vi "real time object finder single cam 4 way v2.0 EJA 09 16 2016.vi"() -> ()   [LabVIEW 2011]
doc: "The Low-Level Grab VI acquires images continuously and displays the images in an image control using low-level acquisition VIs. A grab is appropriate for high-speed applications in which you need to process only one image at a time."
uses:
  <vilib>/userdefined/High Color/IMAQdx.ctl
  <vilib>/vision/driver/IMAQdx.llb/IMAQdx Buffer Number Mode.ctl
  <vilib>/Utility/file.llb/Write To Spreadsheet File (DBL).vi
  <vilib>/vision/driver/NI_Vision_Acquisition_Software.lvlib
  resource/objmgr/imaqdx.rc
  <vilib>/Analysis/NI_AALBase.lvlib
panel:
  in  "Rectangle":T1
  in  "fish size":i32=200
  out "y position histogram":T2(graph)={"X Values"=[105.75, 139.25, 172.75, 206.25, 239.75, 273.25, 306.75, 340.25, 373.75, 407.25], "Histogram: h(x)"=[42, 48, 50, 100, 118, 231, 514, 357, 278, 63]}
  out "x position histogram":T2(graph)={"X Values"=[76.55, 127.65, 178.75, 229.85, 280.95, 332.05, 383.15, 434.25, 485.35, 536.45], "Histogram: h(x)"=[290, 347, 167, 210, 194, 230, 130, 100, 97, 36]}
  in  "histogram \nbins":i32=10
  in  "always save\non stop\nimaging":bool=TRUE
  in  "acquisition \ntime (s)":i32=60
  in  "save for a \ndesignated \nperiod":bool=TRUE
  out "trajectory":cluster{i32[], i32[]}(graph)
  in  "save\nlast\nimage":bool=TRUE
  in  "stop no save":bool
  out "date stub assigned":string="_2016Y_09M_16D_16h_23m_14s"
  in  "Acquire\ndata":bool
  in  "Experimental stub":string="danio01_test"
  out "Saving":bool
  in  "save data":bool
  in  "save path":path=path "E:/danio_tracking_2016/danio01_09_14_2016"
  in  "number\nformat (%.6f)":string="%.6f"
  in  "Marker\nText color":u32(colorbox)=16711680
  out "Multiplot":cluster{cluster{dbl, i32}[]}[](graph)=[{[{0.0, 251}, {0.034, 257}, {0.067, 266}, {0.1, 275}, {0.133, 283}, {0.167, 294}, {0.201, 308}, {0.234, 321}, {0.267, 332}, {0.3, 340}, {0.333, 346}, {0.367, 349}, {0.401, 351}, {0.434, 351}, {0.467, 350}, {0.5, 349}, {0.534, 350}, {0.567, 351}, {0.601, 352}, {0.634, 351}, {0.667, 351}, {0.701, 351}, {0.734, 350}, {0.767, 346}, {0.8, 343}, {0.833, 337}, {0.867, 331}, {0.901, 326}, {0.934, 322}, {0.967, 317}, {1.0, 314}, {1.034, 309}, {1.067, 304}, {1.1, 301}, {1.134, 298}, {1.167, 295}, {1.201, 291}, {1.234, 287}, {1.267, 282}, {1.3, 276}, {1.333, 269}, {1.367, 262}, {1.401, 258}, {1.434, 255}, {1.467, 252}, {1.5, 247}, {1.534, 244}, {1.567, 241}, {1.6, 238}, {1.633, 235}, {1.666, 232}, {1.701, 229}, {1.734, 227}, {1.767, 225}, {1.8, 222}, {1.833, 221}, {1.867, 220}, {1.9, 220}, {1.933, 220}, {1.967, 218}, {2.0, 219}, {2.034, 219}, {2.067, 217}, {2.1, 215}, {2.133, 216}, {2.166, 217}, {2.201, 220}, {2.234, 227}, {2.267, 238}, {2.3, 250}, {2.333, 261}, {2.367, 274}, {2.4, 283}, {2.434, 288}, {2.467, 294}, {2.5, 297}, {2.534, 297}, {2.567, 299}, {2.6, 302}, {2.633, 306}, {2.666, 313}, {2.701, 321}, {2.734, 330}, {2.767, 339}, {2.8, 348}, {2.833, 355}, {2.867, 364}, {2.901, 372}, {2.934, 380}, {2.967, 388}, {3.0, 395}, {3.034, 404}, {3.067, 412}, {3.101, 419}, {3.134, 427}, {3.167, 433}, {3.201, 441}, {3.234, 447}, {3.267, 453}, {3.3, 459}, {3.333, 463}, {3.368, 468}, {3.401, 472}, {3.434, 477}, {3.467, 483}, {3.5, 490}, {3.534, 496}, {3.567, 505}, {3.6, 512}, {3.634, 516}, {3.667, 521}, {3.701, 524}, {3.734, 524}, {3.767, 522}, {3.8, 521}, {3.833, 518}, {3.868, 513}, {3.901, 509}, {3.934, 504}, {3.967, 499}, {4.0, 495}, {4.034, 489}, {4.068, 482}, {4.101, 478}, {4.134, 476}, {4.167, 478}, {4.201, 483}, {4.234, 488}, {4.267, 493}, {4.3, 498}, {4.333, 500}, {4.367, 501}, {4.4, 499}, {4.434, 493}, {4.467, 485}, {4.5, 476}, {4.534, 465}, {4.567, 455}, {4.6, 443}, {4.633, 430}, {4.667, 418}, {4.701, 408}, {4.734, 399}, {4.767, 390}, {4.8, 379}, {4.833, 368}, {4.867, 360}, {4.9, 351}, {4.933, 342}, {4.966, 331}, {5.0, 321}, {5.034, 313}, {5.067, 305}, {5.1, 297}, {5.133, 290}, {5.166, 282}, {5.2, 275}, {5.234, 269}, {5.267, 262}, {5.3, 256}, {5.333, 249}, {5.367, 242}, {5.4, 238}, {5.433, 232}, {5.467, 228}, {5.5, 223}, {5.534, 221}, {5.567, 217}, {5.6, 212}, {5.633, 207}, {5.666, 200}, {5.7, 194}, {5.733, 191}, {5.767, 187}, {5.8, 183}, {5.833, 178}, {5.867, 173}, {5.9, 167}, {5.933, 161}, {5.967, 155}, {6.0, 149}, {6.034, 142}, {6.067, 136}, {6.1, 131}, {6.133, 127}, {6.166, 123}, {6.2, 121}, {6.233, 121}, {6.266, 120}, {6.299, 122}, {6.333, 124}, {6.367, 128}, {6.4, 135}, {6.433, 144}, {6.467, 155}, {6.5, 166}, {6.534, 177}, {6.567, 189}, {6.6, 202}, {6.633, 218}, {6.666, 233}, {6.701, 246}, {6.734, 255}, {6.767, 259}, {6.8, 259}, {6.833, 257}, {6.867, 254}, {6.901, 255}, {6.934, 261}, {6.967, 273}, {7.0, 290}, {7.034, 308}, {7.067, 325}, {7.101, 338}, {7.134, 350}, {7.167, 358}, {7.201, 367}, {7.234, 377}, {7.267, 386}, {7.301, 397}, {7.334, 407}, {7.368, 418}, {7.401, 428}, {7.434, 438}, {7.467, 449}, {7.5, 459}, {7.534, 467}, {7.568, 474}, {7.601, 481}, {7.634, 487}, {7.667, 492}, {7.701, 499}, {7.734, 506}, {7.767, 511}, {7.801, 515}, {7.834, 522}, {7.868, 530}, {7.901, 538}, {7.934, 540}, {7.967, 540}, {8.0, 538}, {8.034, 532}, {8.068, 521}, {8.101, 506}, {8.134, 493}, {8.167, 480}, {8.201, 469}, {8.234, 458}, {8.268, 447}, {8.301, 437}, {8.334, 425}, {8.368, 414}, {8.401, 403}, {8.434, 390}, {8.467, 378}, {8.5, 366}, {8.534, 356}, {8.568, 345}, {8.601, 333}, {8.634, 319}, {8.667, 309}, {8.701, 304}, {8.734, 300}, {8.767, 294}, {8.8, 285}, {8.833, 274}, {8.867, 263}, {8.901, 252}, {8.934, 242}, {8.967, 232}, {9.0, 220}, {9.034, 211}, {9.067, 200}, {9.1, 192}, {9.133, 185}, {9.167, 176}, {9.201, 168}, {9.234, 162}, {9.267, 157}, {9.3, 149}, {9.333, 142}, {9.367, 137}, {9.4, 135}, {9.433, 136}, {9.467, 140}, {9.5, 143}, {9.534, 144}, {9.567, 145}, {9.6, 146}, {9.633, 146}, {9.666, 145}, {9.701, 138}, {9.734, 133}, {9.767, 139}, {9.8, 146}, {9.833, 149}, {9.867, 149}, {9.9, 147}, {9.934, 147}, {9.967, 146}, {10.0, 144}, {10.034, 140}, {10.067, 140}, {10.1, 144}, {10.133, 150}, {10.167, 154}, {10.201, 157}, {10.234, 155}, {10.267, 156}, {10.3, 157}, {10.333, 157}, {10.367, 159}, {10.4, 160}, {10.433, 162}, {10.467, 166}, {10.5, 171}, {10.534, 178}, {10.567, 188}, {10.6, 198}, {10.633, 207}, {10.667, 213}, {10.701, 216}, {10.734, 219}, {10.767, 221}, {10.8, 226}, {10.833, 232}, {10.867, 240}, {10.901, 250}, {10.934, 259}, {10.967, 268}, {11.0, 275}, {11.034, 281}, {11.067, 288}, {11.101, 296}, {11.134, 308}, {11.167, 319}, {11.201, 331}, {11.234, 343}, {11.267, 353}, {11.3, 362}, {11.333, 372}, {11.368, 381}, {11.401, 392}, {11.434, 401}, {11.467, 409}, {11.5, 415}, {11.535, 420}, {11.568, 427}, {11.601, 436}, {11.634, 442}, {11.667, 449}, {11.701, 459}, {11.734, 468}, {11.768, 477}, {11.8, 487}, {11.834, 496}, {11.868, 502}, {11.901, 507}, {11.934, 511}, {11.967, 515}, {12.0, 523}, {12.034, 532}, {12.067, 540}, {12.101, 549}, {12.134, 556}, {12.167, 561}, {12.201, 562}, {12.234, 561}, {12.267, 558}, {12.3, 552}, {12.334, 546}, {12.368, 538}, {12.401, 528}, {12.434, 520}, {12.467, 513}, {12.5, 507}, {12.535, 500}, {12.568, 494}, {12.601, 489}, {12.634, 486}, {12.667, 484}, {12.701, 483}, {12.735, 480}, {12.768, 477}, {12.801, 476}, {12.834, 475}, {12.868, 473}, {12.901, 469}, {12.934, 463}, {12.967, 457}, {13.0, 450}, {13.035, 440}, {13.068, 429}, {13.101, 418}, {13.134, 409}, {13.167, 403}, {13.201, 401}, {13.234, 400}, {13.268, 400}, {13.301, 399}, {13.334, 395}, {13.368, 390}, {13.401, 383}, {13.434, 375}, {13.467, 364}, {13.5, 354}, {13.534, 346}, {13.567, 337}, {13.6, 327}, {13.634, 316}, {13.667, 307}, {13.701, 300}, {13.734, 293}, {13.767, 285}, {13.8, 279}, {13.833, 276}, {13.867, 273}, {13.901, 267}, {13.934, 261}, {13.967, 256}, {14.0, 251}, {14.034, 245}, {14.067, 239}, {14.1, 233}, {14.133, 224}, {14.166, 215}, {14.201, 207}, {14.234, 200}, {14.267, 193}, {14.3, 185}, {14.333, 177}, {14.367, 171}, {14.4, 164}, {14.433, 157}, {14.467, 152}, {14.5, 148}, {14.534, 142}, {14.567, 137}, {14.6, 134}, {14.633, 132}, {14.666, 130}, {14.7, 128}, {14.734, 126}, {14.767, 128}, {14.8, 130}, {14.833, 131}, {14.867, 134}, {14.9, 138}, {14.934, 143}, {14.967, 147}, {15.0, 152}, {15.034, 159}, {15.067, 169}, {15.1, 180}, {15.133, 194}, {15.167, 207}, {15.201, 220}, {15.234, 233}, {15.267, 247}, {15.3, 264}, {15.334, 282}, {15.368, 298}, {15.401, 314}, {15.434, 331}, {15.467, 346}, {15.5, 359}, {15.535, 371}, {15.568, 382}, {15.601, 394}, {15.634, 406}, {15.667, 416}, {15.701, 427}, {15.735, 438}, {15.768, 443}, {15.801, 444}, {15.834, 443}, {15.868, 435}, {15.901, 424}, {15.934, 412}, {15.967, 397}, {16.001, 382}, {16.035, 369}, {16.068, 358}, {16.101, 348}, {16.134, 338}, {16.167, 324}, {16.201, 311}, {16.234, 298}, {16.267, 286}, {16.3, 275}, {16.334, 265}, {16.368, 258}, {16.401, 252}, {16.434, 251}, {16.467, 254}, {16.5, 262}, {16.534, 274}, {16.568, 289}, {16.601, 303}, {16.634, 318}, {16.667, 331}, {16.701, 339}, {16.734, 345}, {16.768, 349}, {16.801, 350}, {16.834, 351}, {16.868, 353}, {16.901, 356}, {16.934, 358}, {16.968, 358}, {17.001, 358}, {17.035, 359}, {17.068, 361}, {17.101, 365}, {17.134, 370}, {17.167, 377}, {17.201, 388}, {17.235, 401}, {17.268, 413}, {17.301, 423}, {17.334, 433}, {17.368, 441}, {17.401, 446}, {17.435, 453}, {17.468, 457}, {17.501, 462}, {17.535, 467}, {17.568, 472}, {17.601, 477}, {17.634, 479}, {17.667, 481}, {17.701, 481}, {17.735, 482}, {17.768, 481}, {17.801, 477}, {17.834, 473}, {17.868, 466}, {17.901, 458}, {17.934, 449}, {17.968, 436}, {18.001, 419}, {18.035, 402}, {18.068, 383}, {18.101, 366}, {18.134, 350}, {18.167, 334}, {18.201, 321}, {18.234, 308}, {18.267, 295}, {18.301, 285}, {18.334, 274}, {18.368, 268}, {18.401, 264}, {18.434, 264}, {18.467, 267}, {18.5, 275}, {18.534, 281}, {18.568, 287}, {18.601, 292}, {18.634, 296}, {18.667, 301}, {18.701, 309}, {18.734, 318}, {18.768, 327}, {18.801, 339}, {18.834, 354}, {18.868, 369}, {18.901, 381}, {18.935, 393}, {18.968, 403}, {19.001, 411}, {19.035, 417}, {19.068, 424}, {19.101, 430}, {19.134, 438}, {19.167, 449}, {19.201, 461}, {19.235, 474}, {19.268, 484}, {19.301, 489}, {19.334, 489}, {19.368, 483}, {19.401, 472}, {19.435, 460}, {19.468, 447}, {19.501, 433}, {19.535, 418}, {19.568, 401}, {19.601, 384}, {19.634, 371}, {19.667, 364}, {19.701, 362}, {19.735, 357}, {19.768, 353}, {19.801, 350}, {19.834, 349}, {19.868, 348}, {19.901, 347}, {19.934, 347}, {19.967, 347}, {20.001, 346}, {20.035, 343}, {20.068, 341}, {20.101, 339}, {20.134, 336}, {20.167, 334}, {20.201, 331}, {20.235, 325}, {20.268, 322}, {20.301, 322}, {20.334, 321}, {20.368, 322}, {20.401, 325}, {20.434, 327}, {20.468, 331}, {20.501, 333}, {20.535, 335}, {20.568, 336}, {20.601, 336}, {20.634, 336}, {20.667, 338}, {20.701, 338}, {20.735, 335}, {20.768, 334}, {20.801, 335}, {20.834, 335}, {20.868, 336}, {20.901, 340}, {20.934, 344}, {20.968, 346}, {21.001, 345}, {21.035, 346}, {21.068, 346}, {21.101, 345}, {21.134, 345}, {21.167, 345}, {21.201, 349}, {21.235, 356}, {21.268, 363}, {21.301, 367}, {21.334, 372}, {21.368, 375}, {21.401, 376}, {21.434, 377}, {21.468, 381}, {21.501, 388}, {21.535, 392}, {21.568, 397}, {21.601, 403}, {21.634, 408}, {21.667, 409}, {21.701, 409}, {21.734, 407}, {21.768, 404}, {21.801, 400}, {21.834, 393}, {21.868, 381}, {21.901, 370}, {21.934, 359}, {21.967, 349}, {22.0, 339}, {22.034, 329}, {22.068, 321}, {22.101, 311}, {22.134, 303}, {22.167, 296}, {22.201, 290}, {22.234, 284}, {22.267, 279}, {22.3, 275}, {22.333, 270}, {22.368, 265}, {22.401, 259}, {22.434, 254}, {22.467, 250}, {22.5, 245}, {22.534, 240}, {22.567, 240}, {22.601, 238}, {22.634, 233}, {22.667, 229}, {22.701, 225}, {22.734, 223}, {22.767, 220}, {22.8, 218}, {22.834, 216}, {22.868, 212}, {22.901, 207}, {22.934, 204}, {22.967, 199}, {23.0, 194}, {23.034, 191}, {23.067, 188}, {23.1, 186}, {23.134, 185}, {23.167, 188}, {23.201, 196}, {23.234, 205}, {23.267, 217}, {23.3, 230}, {23.334, 242}, {23.368, 257}, {23.401, 270}, {23.434, 284}, {23.467, 299}, {23.5, 314}, {23.535, 328}, {23.568, 341}, {23.601, 351}, {23.634, 357}, {23.667, 359}, {23.701, 361}, {23.735, 364}, {23.768, 366}, {23.801, 369}, {23.834, 371}, {23.868, 373}, {23.901, 376}, {23.934, 380}, {23.968, 386}, {24.001, 393}, {24.035, 400}, {24.068, 407}, {24.101, 413}, {24.134, 418}, {24.168, 420}, {24.201, 424}, {24.235, 425}, {24.268, 425}, {24.301, 426}, {24.334, 426}, {24.368, 425}, {24.402, 426}, {24.435, 425}, {24.468, 423}, {24.501, 419}, {24.535, 415}, {24.568, 410}, {24.601, 404}, {24.634, 398}, {24.668, 391}, {24.701, 384}, {24.735, 380}, {24.768, 379}, {24.801, 379}, {24.834, 377}, {24.868, 375}, {24.901, 372}, {24.935, 367}, {24.968, 363}, {25.001, 358}, {25.035, 354}, {25.068, 349}, {25.101, 344}, {25.134, 338}, {25.168, 333}, {25.201, 331}, {25.235, 329}, {25.268, 325}, {25.301, 322}, {25.334, 318}, {25.368, 316}, {25.401, 315}, {25.434, 314}, {25.468, 313}, {25.501, 311}, {25.535, 310}, {25.568, 307}, {25.601, 303}, {25.634, 299}, {25.667, 295}, {25.701, 291}, {25.735, 286}, {25.768, 283}, {25.801, 279}, {25.834, 275}, {25.868, 269}, {25.901, 265}, {25.934, 263}, {25.967, 261}, {26.001, 258}, {26.035, 255}, {26.068, 254}, {26.101, 252}, {26.134, 251}, {26.167, 247}, {26.201, 242}, {26.234, 239}, {26.268, 237}, {26.301, 235}, {26.334, 232}, {26.368, 228}, {26.401, 223}, {26.434, 219}, {26.467, 215}, {26.5, 211}, {26.535, 207}, {26.568, 205}, {26.601, 202}, {26.634, 198}, {26.667, 195}, {26.701, 190}, {26.734, 185}, {26.767, 181}, {26.801, 176}, {26.834, 172}, {26.868, 169}, {26.901, 164}, {26.934, 158}, {26.967, 154}, {27.0, 151}, {27.035, 148}, {27.068, 144}, {27.101, 141}, {27.134, 137}, {27.167, 134}, {27.201, 132}, {27.234, 131}, {27.267, 130}, {27.3, 130}, {27.334, 129}, {27.368, 127}, {27.401, 123}, {27.434, 120}, {27.467, 117}, {27.5, 112}, {27.534, 108}, {27.567, 104}, {27.6, 99}, {27.634, 94}, {27.667, 90}, {27.701, 88}, {27.734, 85}, {27.767, 82}, {27.8, 79}, {27.833, 78}, {27.868, 78}, {27.901, 77}, {27.934, 76}, {27.967, 76}, {28.0, 78}, {28.034, 78}, {28.067, 77}, {28.1, 74}, {28.134, 74}, {28.167, 74}, {28.201, 74}, {28.234, 74}, {28.267, 75}, {28.3, 75}, {28.333, 74}, {28.368, 74}, {28.401, 74}, {28.434, 74}, {28.467, 76}, {28.5, 79}, {28.534, 84}, {28.567, 91}, {28.6, 99}, {28.634, 108}, {28.667, 113}, {28.701, 117}, {28.734, 122}, {28.767, 126}, {28.801, 129}, {28.834, 133}, {28.868, 135}, {28.901, 136}, {28.934, 134}, {28.967, 131}, {29.0, 129}, {29.034, 127}, {29.068, 124}, {29.101, 119}, {29.134, 114}, {29.167, 109}, {29.201, 102}, {29.234, 95}, {29.267, 90}, {29.3, 84}, {29.333, 76}, {29.368, 72}, {29.401, 73}, {29.434, 71}, {29.467, 69}, {29.5, 67}, {29.534, 66}, {29.567, 64}, {29.601, 64}, {29.634, 66}, {29.667, 68}, {29.701, 70}, {29.734, 72}, {29.767, 76}, {29.8, 78}, {29.834, 80}, {29.868, 82}, {29.901, 87}, {29.934, 89}, {29.967, 93}, {30.0, 97}, {30.034, 98}, {30.068, 99}, {30.101, 100}, {30.134, 103}, {30.167, 109}, {30.201, 116}, {30.234, 123}, {30.267, 129}, {30.301, 134}, {30.334, 138}, {30.368, 142}, {30.401, 147}, {30.434, 153}, {30.467, 158}, {30.5, 165}, {30.535, 172}, {30.568, 178}, {30.601, 182}, {30.634, 185}, {30.667, 186}, {30.701, 186}, {30.735, 183}, {30.768, 177}, {30.801, 170}, {30.834, 164}, {30.868, 158}, {30.901, 151}, {30.934, 142}, {30.967, 134}, {31.0, 128}, {31.034, 125}, {31.067, 121}, {31.101, 114}, {31.134, 108}, {31.167, 105}, {31.201, 103}, {31.234, 101}, {31.267, 99}, {31.3, 97}, {31.334, 95}, {31.368, 92}, {31.401, 88}, {31.434, 85}, {31.467, 82}, {31.5, 81}, {31.534, 79}, {31.567, 77}, {31.601, 75}, {31.634, 74}, {31.667, 72}, {31.701, 71}, {31.734, 71}, {31.767, 71}, {31.8, 74}, {31.833, 80}, {31.868, 84}, {31.901, 90}, {31.934, 96}, {31.967, 101}, {32.0, 107}, {32.034, 111}, {32.068, 115}, {32.101, 121}, {32.134, 126}, {32.167, 131}, {32.201, 136}, {32.234, 143}, {32.267, 149}, {32.301, 154}, {32.334, 157}, {32.368, 160}, {32.401, 162}, {32.434, 163}, {32.467, 164}, {32.5, 165}, {32.535, 166}, {32.568, 167}, {32.601, 168}, {32.634, 169}, {32.667, 167}, {32.701, 163}, {32.734, 158}, {32.768, 152}, {32.801, 147}, {32.834, 140}, {32.868, 133}, {32.901, 126}, {32.934, 122}, {32.967, 120}, {33.0, 116}, {33.035, 113}, {33.068, 110}, {33.101, 108}, {33.134, 105}, {33.167, 102}, {33.201, 101}, {33.234, 100}, {33.267, 97}, {33.301, 95}, {33.334, 93}, {33.368, 90}, {33.401, 89}, {33.434, 85}, {33.467, 82}, {33.5, 82}, {33.535, 81}, {33.568, 79}, {33.601, 79}, {33.634, 81}, {33.667, 83}, {33.701, 86}, {33.734, 89}, {33.768, 93}, {33.801, 96}, {33.834, 97}, {33.868, 98}, {33.901, 100}, {33.934, 99}, {33.967, 100}, {34.0, 104}, {34.035, 109}, {34.068, 115}, {34.101, 122}, {34.134, 130}, {34.167, 137}, {34.201, 139}, {34.234, 140}, {34.268, 142}, {34.301, 148}, {34.334, 153}, {34.368, 162}, {34.401, 172}, {34.434, 180}, {34.467, 186}, {34.501, 188}, {34.535, 187}, {34.568, 184}, {34.601, 180}, {34.634, 176}, {34.667, 171}, {34.701, 164}, {34.735, 158}, {34.768, 152}, {34.801, 147}, {34.834, 142}, {34.868, 140}, {34.901, 141}, {34.934, 143}, {34.967, 145}, {35.0, 145}, {35.035, 144}, {35.068, 143}, {35.101, 138}, {35.134, 131}, {35.167, 123}, {35.201, 116}, {35.234, 111}, {35.268, 105}, {35.301, 100}, {35.334, 98}, {35.368, 96}, {35.401, 95}, {35.434, 95}, {35.467, 95}, {35.5, 96}, {35.534, 95}, {35.568, 93}, {35.601, 94}, {35.634, 95}, {35.667, 95}, {35.701, 94}, {35.734, 91}, {35.767, 91}, {35.801, 90}, {35.834, 88}, {35.868, 85}, {35.901, 83}, {35.934, 82}, {35.967, 84}, {36.0, 87}, {36.035, 93}, {36.068, 101}, {36.101, 108}, {36.134, 115}, {36.167, 121}, {36.201, 126}, {36.234, 129}, {36.268, 133}, {36.301, 135}, {36.334, 135}, {36.368, 136}, {36.401, 137}, {36.434, 137}, {36.468, 133}, {36.501, 132}, {36.535, 132}, {36.568, 131}, {36.601, 130}, {36.634, 131}, {36.667, 133}, {36.701, 133}, {36.734, 133}, {36.768, 132}, {36.801, 130}, {36.834, 129}, {36.868, 129}, {36.901, 129}, {36.934, 129}, {36.967, 126}, {37.001, 122}, {37.035, 118}, {37.068, 114}, {37.101, 109}, {37.134, 102}, {37.167, 96}, {37.201, 94}, {37.234, 92}, {37.268, 91}, {37.301, 91}, {37.334, 90}, {37.368, 89}, {37.401, 86}, {37.434, 81}, {37.467, 77}, {37.5, 73}, {37.535, 68}, {37.568, 64}, {37.601, 59}, {37.634, 56}, {37.667, 54}, {37.701, 54}, {37.734, 53}, {37.768, 51}, {37.801, 51}, {37.834, 52}, {37.868, 53}, {37.901, 55}, {37.934, 56}, {37.967, 58}, {38.0, 61}, {38.035, 64}, {38.068, 65}, {38.101, 68}, {38.134, 72}, {38.167, 77}, {38.201, 80}, {38.234, 84}, {38.268, 88}, {38.301, 93}, {38.334, 96}, {38.368, 97}, {38.401, 97}, {38.434, 100}, {38.467, 103}, {38.5, 106}, {38.535, 110}, {38.568, 115}, {38.601, 124}, {38.634, 131}, {38.667, 136}, {38.701, 139}, {38.735, 141}, {38.768, 141}, {38.801, 143}, {38.834, 145}, {38.868, 149}, {38.901, 153}, {38.934, 156}, {38.967, 156}, {39.001, 155}, {39.035, 153}, {39.068, 151}, {39.101, 147}, {39.134, 141}, {39.167, 133}, {39.201, 126}, {39.234, 121}, {39.268, 119}, {39.301, 119}, {39.334, 116}, {39.368, 112}, {39.401, 109}, {39.434, 106}, {39.467, 102}, {39.5, 96}, {39.534, 92}, {39.568, 88}, {39.601, 83}, {39.634, 79}, {39.667, 75}, {39.701, 70}, {39.734, 68}, {39.767, 64}, {39.801, 60}, {39.834, 60}, {39.868, 63}, {39.901, 64}, {39.934, 66}, {39.967, 69}, {40.0, 74}, {40.034, 79}, {40.068, 82}, {40.101, 85}, {40.134, 87}, {40.167, 90}, {40.201, 92}, {40.234, 96}, {40.268, 100}, {40.301, 104}, {40.334, 109}, {40.368, 114}, {40.401, 120}, {40.434, 126}, {40.468, 131}, {40.501, 134}, {40.535, 138}, {40.568, 141}, {40.601, 144}, {40.634, 145}, {40.667, 146}, {40.701, 147}, {40.735, 146}, {40.768, 144}, {40.801, 141}, {40.834, 139}, {40.868, 138}, {40.901, 137}, {40.935, 135}, {40.968, 134}, {41.001, 132}, {41.035, 131}, {41.068, 130}, {41.101, 128}, {41.134, 125}, {41.167, 122}, {41.201, 120}, {41.234, 117}, {41.268, 113}, {41.301, 109}, {41.334, 107}, {41.368, 105}, {41.401, 104}, {41.434, 102}, {41.467, 98}, {41.501, 95}, {41.535, 93}, {41.568, 91}, {41.601, 90}, {41.634, 88}, {41.667, 86}, {41.701, 85}, {41.734, 83}, {41.767, 81}, {41.801, 80}, {41.834, 79}, {41.868, 79}, {41.901, 81}, {41.934, 84}, {41.967, 88}, {42.001, 93}, {42.035, 97}, {42.068, 103}, {42.101, 109}, {42.134, 115}, {42.167, 121}, {42.201, 125}, {42.235, 129}, {42.268, 131}, {42.301, 132}, {42.334, 132}, {42.368, 133}, {42.401, 136}, {42.434, 138}, {42.468, 138}, {42.501, 139}, {42.535, 144}, {42.568, 147}, {42.601, 150}, {42.634, 152}, {42.668, 152}, {42.701, 153}, {42.735, 152}, {42.768, 151}, {42.801, 149}, {42.834, 146}, {42.868, 144}, {42.901, 139}, {42.934, 134}, {42.968, 130}, {43.001, 125}, {43.035, 120}, {43.068, 115}, {43.101, 110}, {43.134, 104}, {43.167, 100}, {43.201, 97}, {43.235, 93}, {43.268, 90}, {43.301, 88}, {43.334, 85}, {43.368, 83}, {43.401, 80}, {43.434, 78}, {43.467, 77}, {43.501, 76}, {43.535, 74}, {43.568, 73}, {43.601, 75}, {43.634, 75}, {43.667, 74}, {43.701, 73}, {43.734, 74}, {43.768, 74}, {43.801, 74}, {43.834, 74}, {43.868, 74}, {43.901, 76}, {43.934, 76}, {43.967, 75}, {44.001, 76}, {44.035, 77}, {44.068, 78}, {44.101, 82}, {44.134, 87}, {44.167, 93}, {44.201, 100}, {44.235, 108}, {44.268, 114}, {44.301, 118}, {44.334, 121}, {44.368, 122}, {44.401, 122}, {44.434, 122}, {44.468, 121}, {44.501, 119}, {44.535, 115}, {44.568, 113}, {44.601, 112}, {44.634, 113}, {44.667, 116}, {44.701, 119}, {44.735, 121}, {44.768, 121}, {44.801, 118}, {44.834, 114}, {44.868, 108}, {44.901, 102}, {44.934, 98}, {44.967, 94}, {45.001, 90}, {45.035, 85}, {45.068, 78}, {45.101, 70}, {45.134, 65}, {45.167, 62}, {45.201, 61}, {45.234, 62}, {45.267, 63}, {45.301, 65}, {45.334, 68}, {45.368, 73}, {45.401, 80}, {45.434, 88}, {45.467, 94}, {45.501, 100}, {45.535, 106}, {45.568, 111}, {45.601, 117}, {45.634, 122}, {45.667, 128}, {45.701, 135}, {45.735, 140}, {45.768, 141}, {45.801, 138}, {45.834, 134}, {45.868, 128}, {45.901, 123}, {45.934, 121}, {45.967, 118}, {46.0, 114}, {46.034, 109}, {46.068, 105}, {46.101, 101}, {46.134, 98}, {46.167, 95}, {46.201, 91}, {46.234, 88}, {46.268, 85}, {46.301, 81}, {46.334, 81}, {46.368, 79}, {46.401, 77}, {46.434, 75}, {46.467, 71}, {46.5, 69}, {46.535, 70}, {46.568, 71}, {46.601, 71}, {46.634, 72}, {46.667, 75}, {46.701, 77}, {46.734, 79}, {46.768, 84}, {46.801, 90}, {46.834, 96}, {46.868, 101}, {46.901, 104}, {46.934, 107}, {46.968, 110}, {47.001, 110}, {47.035, 111}, {47.068, 113}, {47.101, 117}, {47.134, 121}, {47.168, 126}, {47.201, 131}, {47.235, 135}, {47.268, 140}, {47.301, 145}, {47.334, 148}, {47.368, 149}, {47.402, 149}, {47.435, 150}, {47.468, 154}, {47.501, 157}, {47.535, 161}, {47.568, 165}, {47.601, 170}, {47.634, 174}, {47.668, 178}, {47.701, 182}, {47.735, 186}, {47.768, 190}, {47.801, 192}, {47.834, 194}, {47.868, 197}, {47.901, 200}, {47.934, 204}, {47.968, 207}, {48.001, 209}, {48.035, 212}, {48.068, 216}, {48.101, 220}, {48.134, 226}, {48.168, 232}, {48.201, 238}, {48.235, 245}, {48.268, 253}, {48.301, 259}, {48.334, 265}, {48.368, 270}, {48.402, 273}, {48.435, 278}, {48.468, 284}, {48.501, 290}, {48.535, 296}, {48.568, 303}, {48.601, 312}, {48.635, 320}, {48.668, 329}, {48.701, 337}, {48.735, 345}, {48.768, 354}, {48.801, 362}, {48.835, 370}, {48.868, 379}, {48.902, 387}, {48.935, 396}, {48.968, 403}, {49.001, 411}, {49.035, 420}, {49.068, 427}, {49.102, 433}, {49.135, 439}, {49.168, 442}, {49.201, 446}, {49.235, 449}, {49.268, 452}, {49.302, 456}, {49.335, 460}, {49.368, 465}, {49.402, 471}, {49.435, 477}, {49.468, 484}, {49.501, 489}, {49.535, 494}, {49.569, 498}, {49.602, 499}, {49.635, 498}, {49.668, 496}, {49.701, 492}, {49.735, 486}, {49.769, 480}, {49.802, 474}, {49.835, 469}, {49.868, 466}, {49.902, 460}, {49.935, 453}, {49.969, 446}, {50.002, 441}, {50.035, 436}, {50.069, 430}, {50.102, 423}, {50.135, 415}, {50.168, 409}, {50.201, 403}, {50.235, 396}, {50.269, 390}, {50.301, 385}, {50.335, 378}, {50.368, 372}, {50.402, 368}, {50.435, 365}, {50.468, 364}, {50.501, 362}, {50.535, 359}, {50.569, 357}, {50.602, 354}, {50.635, 352}, {50.668, 349}, {50.701, 346}, {50.735, 344}, {50.769, 343}, {50.802, 341}, {50.835, 339}, {50.868, 337}, {50.902, 334}, {50.935, 331}, {50.968, 328}, {51.001, 326}, {51.035, 324}, {51.069, 322}, {51.102, 321}, {51.135, 321}, {51.168, 320}, {51.201, 319}, {51.235, 320}, {51.269, 321}, {51.302, 320}, {51.335, 320}, {51.368, 319}, {51.402, 319}, {51.435, 318}, {51.468, 318}, {51.502, 319}, {51.535, 319}, {51.569, 320}, {51.602, 321}, {51.635, 321}, {51.668, 320}, {51.701, 318}, {51.735, 314}, {51.768, 309}, {51.802, 302}, {51.835, 297}, {51.868, 294}, {51.902, 290}, {51.935, 284}, {51.968, 280}, {52.001, 275}, {52.035, 270}, {52.069, 267}, {52.102, 262}, {52.135, 258}, {52.168, 256}, {52.201, 256}, {52.235, 256}, {52.268, 254}, {52.301, 251}, {52.335, 249}, {52.368, 246}, {52.402, 242}, {52.435, 239}, {52.468, 237}, {52.501, 238}, {52.535, 241}, {52.568, 245}, {52.602, 250}, {52.635, 256}, {52.668, 263}, {52.701, 271}, {52.735, 276}, {52.768, 282}, {52.802, 290}, {52.835, 297}, {52.868, 303}, {52.902, 309}, {52.935, 314}, {52.968, 319}, {53.002, 323}, {53.035, 326}, {53.069, 328}, {53.102, 329}, {53.135, 329}, {53.168, 328}, {53.201, 327}, {53.236, 326}, {53.269, 324}, {53.302, 321}, {53.335, 317}, {53.368, 310}, {53.402, 303}, {53.435, 299}, {53.468, 295}, {53.502, 294}, {53.535, 294}, {53.569, 292}, {53.602, 290}, {53.635, 288}, {53.668, 287}, {53.701, 285}, {53.735, 282}, {53.769, 277}, {53.802, 271}, {53.835, 265}, {53.868, 260}, {53.902, 257}, {53.935, 255}, {53.968, 253}, {54.001, 250}, {54.035, 248}, {54.069, 245}, {54.101, 244}, {54.135, 243}, {54.168, 240}, {54.201, 237}, {54.235, 234}, {54.268, 230}, {54.302, 226}, {54.335, 222}, {54.368, 218}, {54.402, 214}, {54.435, 210}, {54.468, 208}, {54.501, 206}, {54.535, 202}, {54.568, 199}, {54.601, 196}, {54.635, 193}, {54.668, 190}, {54.701, 189}, {54.735, 189}, {54.768, 188}, {54.802, 187}, {54.834, 188}, {54.868, 192}, {54.902, 194}, {54.935, 197}, {54.968, 201}, {55.001, 207}, {55.035, 213}, {55.069, 221}, {55.102, 228}, {55.135, 235}, {55.168, 242}, {55.201, 247}, {55.235, 251}, {55.268, 252}, {55.302, 251}, {55.335, 251}, {55.368, 250}, {55.402, 250}, {55.435, 253}, {55.468, 255}, {55.501, 257}, {55.535, 258}, {55.569, 257}, {55.602, 256}, {55.635, 253}, {55.668, 251}, {55.701, 247}, {55.735, 242}, {55.768, 236}, {55.802, 230}, {55.835, 223}, {55.868, 216}, {55.902, 208}, {55.935, 202}, {55.968, 198}, {56.001, 192}, {56.035, 187}, {56.068, 184}, {56.102, 181}, {56.135, 178}, {56.168, 176}, {56.201, 175}, {56.235, 173}, {56.268, 170}, {56.301, 166}, {56.335, 161}, {56.368, 156}, {56.402, 151}, {56.435, 148}, {56.468, 145}, {56.501, 143}, {56.535, 143}, {56.568, 145}, {56.602, 147}, {56.635, 150}, {56.668, 156}, {56.701, 163}, {56.735, 170}, {56.769, 177}, {56.802, 185}, {56.835, 190}, {56.868, 195}, {56.902, 201}, {56.935, 205}, {56.968, 211}, {57.001, 216}, {57.035, 219}, {57.069, 222}, {57.102, 224}, {57.135, 227}, {57.168, 231}, {57.201, 236}, {57.235, 241}, {57.269, 247}, {57.302, 254}, {57.335, 260}, {57.368, 265}, {57.402, 269}, {57.435, 273}, {57.469, 277}, {57.502, 278}, {57.535, 278}, {57.569, 277}, {57.602, 274}, {57.635, 272}, {57.668, 270}, {57.701, 265}, {57.735, 258}, {57.769, 251}, {57.802, 247}, {57.835, 242}, {57.868, 237}, {57.902, 232}, {57.935, 228}, {57.968, 226}, {58.001, 226}, {58.043, 227}, {58.069, 230}, {58.102, 237}, {58.135, 245}, {58.168, 252}, {58.201, 259}, {58.235, 265}, {58.268, 272}, {58.302, 277}, {58.335, 281}, {58.368, 284}, {58.402, 289}, {58.435, 294}, {58.468, 297}, {58.501, 303}, {58.535, 309}, {58.569, 314}, {58.602, 320}, {58.635, 325}, {58.668, 330}, {58.701, 338}, {58.744, 346}, {58.769, 351}, {58.802, 354}, {58.835, 353}, {58.868, 349}, {58.902, 346}, {58.935, 340}, {58.969, 332}, {59.007, 326}, {59.035, 318}, {59.069, 309}, {59.102, 301}, {59.135, 292}, {59.168, 284}, {59.201, 277}, {59.236, 271}, {59.269, 264}, {59.302, 260}, {59.335, 258}, {59.368, 255}, {59.402, 251}, {59.435, 245}, {59.468, 239}, {59.502, 234}, {59.535, 229}, {59.569, 223}, {59.602, 217}, {59.635, 212}, {59.668, 211}, {59.701, 209}, {59.735, 208}, {59.769, 207}, {59.802, 205}, {59.835, 203}, {59.868, 200}, {59.902, 198}, {59.935, 197}, {59.968, 196}, {60.001, 195}]}, {[{0.0, 275}, {0.034, 266}, {0.067, 249}, {0.1, 235}, {0.133, 224}, {0.167, 220}, {0.201, 209}, {0.234, 200}, {0.267, 202}, {0.3, 200}, {0.333, 192}, {0.367, 199}, {0.401, 202}, {0.434, 211}, {0.467, 212}, {0.5, 223}, {0.534, 227}, {0.567, 232}, {0.601, 235}, {0.634, 236}, {0.667, 233}, {0.701, 227}, {0.734, 216}, {0.767, 214}, {0.8, 201}, {0.833, 197}, {0.867, 189}, {0.901, 192}, {0.934, 194}, {0.967, 202}, {1.0, 211}, {1.034, 225}, {1.067, 241}, {1.1, 255}, {1.134, 267}, {1.167, 274}, {1.201, 279}, {1.234, 279}, {1.267, 277}, {1.3, 269}, {1.333, 267}, {1.367, 259}, {1.401, 252}, {1.434, 244}, {1.467, 240}, {1.5, 240}, {1.534, 238}, {1.567, 237}, {1.6, 239}, {1.633, 243}, {1.666, 251}, {1.701, 261}, {1.734, 273}, {1.767, 281}, {1.8, 291}, {1.833, 295}, {1.867, 294}, {1.9, 284}, {1.933, 274}, {1.967, 264}, {2.0, 247}, {2.034, 235}, {2.067, 225}, {2.1, 214}, {2.133, 206}, {2.166, 204}, {2.201, 204}, {2.234, 199}, {2.267, 201}, {2.3, 199}, {2.333, 198}, {2.367, 193}, {2.4, 187}, {2.434, 181}, {2.467, 169}, {2.5, 158}, {2.534, 149}, {2.567, 136}, {2.6, 125}, {2.633, 121}, {2.666, 112}, {2.701, 111}, {2.734, 115}, {2.767, 117}, {2.8, 118}, {2.833, 128}, {2.867, 127}, {2.901, 130}, {2.934, 131}, {2.967, 130}, {3.0, 133}, {3.034, 125}, {3.067, 119}, {3.101, 118}, {3.134, 113}, {3.167, 110}, {3.201, 103}, {3.234, 102}, {3.267, 105}, {3.3, 100}, {3.333, 100}, {3.368, 102}, {3.401, 104}, {3.434, 101}, {3.467, 108}, {3.5, 112}, {3.534, 114}, {3.567, 120}, {3.6, 127}, {3.634, 136}, {3.667, 148}, {3.701, 154}, {3.734, 168}, {3.767, 177}, {3.8, 187}, {3.833, 198}, {3.868, 209}, {3.901, 220}, {3.934, 231}, {3.967, 245}, {4.0, 258}, {4.034, 272}, {4.068, 289}, {4.101, 307}, {4.134, 324}, {4.167, 339}, {4.201, 353}, {4.234, 368}, {4.267, 382}, {4.3, 395}, {4.333, 406}, {4.367, 415}, {4.4, 420}, {4.434, 424}, {4.467, 422}, {4.5, 419}, {4.534, 414}, {4.567, 409}, {4.6, 403}, {4.633, 401}, {4.667, 397}, {4.701, 391}, {4.734, 391}, {4.767, 393}, {4.8, 398}, {4.833, 407}, {4.867, 413}, {4.9, 417}, {4.933, 420}, {4.966, 419}, {5.0, 418}, {5.034, 411}, {5.067, 405}, {5.1, 398}, {5.133, 391}, {5.166, 382}, {5.2, 377}, {5.234, 375}, {5.267, 371}, {5.3, 370}, {5.333, 369}, {5.367, 370}, {5.4, 369}, {5.433, 371}, {5.467, 374}, {5.5, 377}, {5.534, 381}, {5.567, 383}, {5.6, 388}, {5.633, 391}, {5.666, 395}, {5.7, 396}, {5.733, 391}, {5.767, 386}, {5.8, 379}, {5.833, 369}, {5.867, 361}, {5.9, 350}, {5.933, 343}, {5.967, 338}, {6.0, 336}, {6.034, 338}, {6.067, 342}, {6.1, 347}, {6.133, 354}, {6.166, 361}, {6.2, 368}, {6.233, 371}, {6.266, 370}, {6.299, 365}, {6.333, 358}, {6.367, 342}, {6.4, 330}, {6.433, 318}, {6.467, 310}, {6.5, 305}, {6.534, 304}, {6.567, 304}, {6.6, 307}, {6.633, 310}, {6.666, 317}, {6.701, 321}, {6.734, 326}, {6.767, 327}, {6.8, 326}, {6.833, 323}, {6.867, 316}, {6.901, 306}, {6.934, 302}, {6.967, 303}, {7.0, 311}, {7.034, 321}, {7.067, 337}, {7.101, 352}, {7.134, 363}, {7.167, 370}, {7.201, 366}, {7.234, 356}, {7.267, 343}, {7.301, 330}, {7.334, 321}, {7.368, 314}, {7.401, 313}, {7.434, 314}, {7.467, 315}, {7.5, 316}, {7.534, 318}, {7.568, 319}, {7.601, 318}, {7.634, 315}, {7.667, 311}, {7.701, 303}, {7.734, 301}, {7.767, 294}, {7.801, 296}, {7.834, 301}, {7.868, 308}, {7.901, 316}, {7.934, 324}, {7.967, 327}, {8.0, 325}, {8.034, 323}, {8.068, 317}, {8.101, 309}, {8.134, 300}, {8.167, 295}, {8.201, 291}, {8.234, 292}, {8.268, 293}, {8.301, 293}, {8.334, 293}, {8.368, 294}, {8.401, 294}, {8.434, 298}, {8.467, 297}, {8.5, 307}, {8.534, 307}, {8.568, 311}, {8.601, 318}, {8.634, 319}, {8.667, 315}, {8.701, 316}, {8.734, 308}, {8.767, 305}, {8.8, 304}, {8.833, 305}, {8.867, 306}, {8.901, 307}, {8.934, 309}, {8.967, 309}, {9.0, 309}, {9.034, 306}, {9.067, 305}, {9.1, 304}, {9.133, 303}, {9.167, 304}, {9.201, 306}, {9.234, 306}, {9.267, 304}, {9.3, 301}, {9.333, 298}, {9.367, 294}, {9.4, 294}, {9.433, 300}, {9.467, 310}, {9.5, 320}, {9.534, 330}, {9.567, 335}, {9.6, 327}, {9.633, 316}, {9.666, 304}, {9.701, 287}, {9.734, 268}, {9.767, 238}, {9.8, 228}, {9.833, 219}, {9.867, 217}, {9.9, 213}, {9.934, 210}, {9.967, 208}, {10.0, 211}, {10.034, 216}, {10.067, 221}, {10.1, 212}, {10.133, 205}, {10.167, 198}, {10.201, 185}, {10.234, 173}, {10.267, 161}, {10.3, 155}, {10.333, 140}, {10.367, 129}, {10.4, 123}, {10.433, 118}, {10.467, 115}, {10.5, 118}, {10.534, 124}, {10.567, 130}, {10.6, 138}, {10.633, 146}, {10.667, 152}, {10.701, 159}, {10.734, 161}, {10.767, 160}, {10.8, 157}, {10.833, 154}, {10.867, 153}, {10.901, 152}, {10.934, 155}, {10.967, 155}, {11.0, 152}, {11.034, 145}, {11.067, 137}, {11.101, 127}, {11.134, 115}, {11.167, 106}, {11.201, 103}, {11.234, 105}, {11.267, 109}, {11.3, 116}, {11.333, 124}, {11.368, 131}, {11.401, 138}, {11.434, 141}, {11.467, 140}, {11.5, 134}, {11.535, 129}, {11.568, 113}, {11.601, 102}, {11.634, 95}, {11.667, 95}, {11.701, 89}, {11.734, 92}, {11.768, 96}, {11.8, 102}, {11.834, 109}, {11.868, 115}, {11.901, 120}, {11.934, 125}, {11.967, 129}, {12.0, 130}, {12.034, 132}, {12.067, 137}, {12.101, 140}, {12.134, 144}, {12.167, 148}, {12.201, 151}, {12.234, 159}, {12.267, 167}, {12.3, 179}, {12.334, 193}, {12.368, 207}, {12.401, 224}, {12.434, 238}, {12.467, 246}, {12.5, 250}, {12.535, 252}, {12.568, 252}, {12.601, 251}, {12.634, 250}, {12.667, 250}, {12.701, 259}, {12.735, 270}, {12.768, 286}, {12.801, 303}, {12.834, 316}, {12.868, 323}, {12.901, 328}, {12.934, 327}, {12.967, 323}, {13.0, 316}, {13.035, 312}, {13.068, 308}, {13.101, 307}, {13.134, 309}, {13.167, 315}, {13.201, 323}, {13.234, 334}, {13.268, 344}, {13.301, 356}, {13.334, 364}, {13.368, 373}, {13.401, 378}, {13.434, 379}, {13.467, 379}, {13.5, 379}, {13.534, 376}, {13.567, 374}, {13.6, 372}, {13.634, 371}, {13.667, 370}, {13.701, 367}, {13.734, 366}, {13.767, 368}, {13.8, 372}, {13.833, 372}, {13.867, 375}, {13.901, 380}, {13.934, 382}, {13.967, 384}, {14.0, 385}, {14.034, 386}, {14.067, 385}, {14.1, 382}, {14.133, 380}, {14.166, 378}, {14.201, 373}, {14.234, 368}, {14.267, 365}, {14.3, 364}, {14.333, 364}, {14.367, 366}, {14.4, 368}, {14.433, 372}, {14.467, 375}, {14.5, 376}, {14.534, 381}, {14.567, 382}, {14.6, 380}, {14.633, 375}, {14.666, 368}, {14.7, 359}, {14.734, 349}, {14.767, 335}, {14.8, 321}, {14.833, 314}, {14.867, 303}, {14.9, 291}, {14.934, 284}, {14.967, 281}, {15.0, 281}, {15.034, 283}, {15.067, 285}, {15.1, 290}, {15.133, 293}, {15.167, 295}, {15.201, 296}, {15.234, 297}, {15.267, 297}, {15.3, 300}, {15.334, 300}, {15.368, 297}, {15.401, 299}, {15.434, 301}, {15.467, 303}, {15.5, 308}, {15.535, 310}, {15.568, 315}, {15.601, 317}, {15.634, 318}, {15.667, 323}, {15.701, 325}, {15.735, 326}, {15.768, 330}, {15.801, 333}, {15.834, 334}, {15.868, 335}, {15.901, 337}, {15.934, 337}, {15.967, 341}, {16.001, 344}, {16.035, 347}, {16.068, 349}, {16.101, 350}, {16.134, 350}, {16.167, 353}, {16.201, 355}, {16.234, 357}, {16.267, 356}, {16.3, 354}, {16.334, 349}, {16.368, 345}, {16.401, 342}, {16.434, 338}, {16.467, 333}, {16.5, 324}, {16.534, 320}, {16.568, 322}, {16.601, 321}, {16.634, 320}, {16.667, 319}, {16.701, 317}, {16.734, 311}, {16.768, 300}, {16.801, 295}, {16.834, 285}, {16.868, 269}, {16.901, 252}, {16.934, 242}, {16.968, 234}, {17.001, 223}, {17.035, 214}, {17.068, 210}, {17.101, 207}, {17.134, 206}, {17.167, 206}, {17.201, 207}, {17.235, 206}, {17.268, 209}, {17.301, 213}, {17.334, 215}, {17.368, 218}, {17.401, 219}, {17.435, 214}, {17.468, 210}, {17.501, 202}, {17.535, 195}, {17.568, 185}, {17.601, 175}, {17.634, 169}, {17.667, 163}, {17.701, 161}, {17.735, 158}, {17.768, 159}, {17.801, 159}, {17.834, 160}, {17.868, 162}, {17.901, 163}, {17.934, 162}, {17.968, 164}, {18.001, 166}, {18.035, 166}, {18.068, 167}, {18.101, 169}, {18.134, 167}, {18.167, 170}, {18.201, 167}, {18.234, 165}, {18.267, 165}, {18.301, 167}, {18.334, 172}, {18.368, 179}, {18.401, 186}, {18.434, 191}, {18.467, 199}, {18.5, 202}, {18.534, 210}, {18.568, 214}, {18.601, 217}, {18.634, 217}, {18.667, 216}, {18.701, 214}, {18.734, 213}, {18.768, 213}, {18.801, 213}, {18.834, 213}, {18.868, 215}, {18.901, 219}, {18.935, 222}, {18.968, 228}, {19.001, 236}, {19.035, 244}, {19.068, 252}, {19.101, 258}, {19.134, 262}, {19.167, 263}, {19.201, 264}, {19.235, 265}, {19.268, 268}, {19.301, 271}, {19.334, 278}, {19.368, 284}, {19.401, 293}, {19.435, 300}, {19.468, 308}, {19.501, 311}, {19.535, 313}, {19.568, 314}, {19.601, 317}, {19.634, 309}, {19.667, 308}, {19.701, 299}, {19.735, 303}, {19.768, 299}, {19.801, 304}, {19.834, 304}, {19.868, 305}, {19.901, 303}, {19.934, 303}, {19.967, 299}, {20.001, 294}, {20.035, 292}, {20.068, 289}, {20.101, 284}, {20.134, 281}, {20.167, 274}, {20.201, 274}, {20.235, 275}, {20.268, 275}, {20.301, 277}, {20.334, 279}, {20.368, 280}, {20.401, 282}, {20.434, 284}, {20.468, 281}, {20.501, 276}, {20.535, 277}, {20.568, 273}, {20.601, 269}, {20.634, 267}, {20.667, 261}, {20.701, 256}, {20.735, 256}, {20.768, 252}, {20.801, 248}, {20.834, 244}, {20.868, 247}, {20.901, 247}, {20.934, 244}, {20.968, 249}, {21.001, 256}, {21.035, 264}, {21.068, 272}, {21.101, 282}, {21.134, 290}, {21.167, 301}, {21.201, 302}, {21.235, 299}, {21.268, 294}, {21.301, 295}, {21.334, 294}, {21.368, 296}, {21.401, 303}, {21.434, 313}, {21.468, 323}, {21.501, 333}, {21.535, 343}, {21.568, 353}, {21.601, 360}, {21.634, 367}, {21.667, 371}, {21.701, 376}, {21.734, 378}, {21.768, 375}, {21.801, 375}, {21.834, 374}, {21.868, 375}, {21.901, 375}, {21.934, 374}, {21.967, 374}, {22.0, 373}, {22.034, 374}, {22.068, 375}, {22.101, 379}, {22.134, 382}, {22.167, 385}, {22.201, 388}, {22.234, 396}, {22.267, 395}, {22.3, 397}, {22.333, 396}, {22.368, 394}, {22.401, 390}, {22.434, 383}, {22.467, 374}, {22.5, 365}, {22.534, 357}, {22.567, 346}, {22.601, 339}, {22.634, 336}, {22.667, 333}, {22.701, 331}, {22.734, 333}, {22.767, 329}, {22.8, 335}, {22.834, 339}, {22.868, 345}, {22.901, 352}, {22.934, 359}, {22.967, 365}, {23.0, 370}, {23.034, 371}, {23.067, 371}, {23.1, 373}, {23.134, 368}, {23.167, 364}, {23.201, 358}, {23.234, 352}, {23.267, 346}, {23.3, 340}, {23.334, 337}, {23.368, 333}, {23.401, 333}, {23.434, 335}, {23.467, 338}, {23.5, 343}, {23.535, 353}, {23.568, 360}, {23.601, 362}, {23.634, 364}, {23.667, 363}, {23.701, 361}, {23.735, 353}, {23.768, 342}, {23.801, 332}, {23.834, 321}, {23.868, 315}, {23.901, 309}, {23.934, 311}, {23.968, 314}, {24.001, 316}, {24.035, 327}, {24.068, 329}, {24.101, 336}, {24.134, 342}, {24.168, 347}, {24.201, 343}, {24.235, 338}, {24.268, 329}, {24.301, 317}, {24.334, 307}, {24.368, 296}, {24.402, 279}, {24.435, 272}, {24.468, 263}, {24.501, 257}, {24.535, 249}, {24.568, 253}, {24.601, 256}, {24.634, 261}, {24.668, 270}, {24.701, 282}, {24.735, 296}, {24.768, 305}, {24.801, 312}, {24.834, 319}, {24.868, 319}, {24.901, 311}, {24.935, 302}, {24.968, 292}, {25.001, 278}, {25.035, 265}, {25.068, 252}, {25.101, 242}, {25.134, 236}, {25.168, 237}, {25.201, 237}, {25.235, 244}, {25.268, 254}, {25.301, 271}, {25.334, 284}, {25.368, 297}, {25.401, 308}, {25.434, 317}, {25.468, 314}, {25.501, 311}, {25.535, 303}, {25.568, 295}, {25.601, 287}, {25.634, 277}, {25.667, 268}, {25.701, 262}, {25.735, 262}, {25.768, 260}, {25.801, 267}, {25.834, 274}, {25.868, 284}, {25.901, 297}, {25.934, 308}, {25.967, 319}, {26.001, 328}, {26.035, 331}, {26.068, 333}, {26.101, 332}, {26.134, 326}, {26.167, 320}, {26.201, 312}, {26.234, 302}, {26.268, 294}, {26.301, 287}, {26.334, 289}, {26.368, 291}, {26.401, 290}, {26.434, 295}, {26.467, 302}, {26.5, 311}, {26.535, 313}, {26.568, 319}, {26.601, 324}, {26.634, 322}, {26.667, 322}, {26.701, 321}, {26.734, 319}, {26.767, 315}, {26.801, 312}, {26.834, 309}, {26.868, 307}, {26.901, 303}, {26.934, 301}, {26.967, 299}, {27.0, 297}, {27.035, 298}, {27.068, 302}, {27.101, 304}, {27.134, 306}, {27.167, 306}, {27.201, 314}, {27.234, 321}, {27.267, 327}, {27.3, 330}, {27.334, 335}, {27.368, 334}, {27.401, 335}, {27.434, 334}, {27.467, 330}, {27.5, 329}, {27.534, 327}, {27.567, 326}, {27.6, 324}, {27.634, 322}, {27.667, 320}, {27.701, 318}, {27.734, 317}, {27.767, 317}, {27.8, 321}, {27.833, 319}, {27.868, 325}, {27.901, 328}, {27.934, 330}, {27.967, 333}, {28.0, 334}, {28.034, 334}, {28.067, 334}, {28.1, 333}, {28.134, 329}, {28.167, 322}, {28.201, 318}, {28.234, 311}, {28.267, 305}, {28.3, 299}, {28.333, 297}, {28.368, 295}, {28.401, 294}, {28.434, 293}, {28.467, 290}, {28.5, 291}, {28.534, 293}, {28.567, 293}, {28.6, 292}, {28.634, 290}, {28.667, 291}, {28.701, 292}, {28.734, 293}, {28.767, 294}, {28.801, 296}, {28.834, 295}, {28.868, 291}, {28.901, 290}, {28.934, 284}, {28.967, 279}, {29.0, 273}, {29.034, 268}, {29.068, 262}, {29.101, 257}, {29.134, 253}, {29.167, 249}, {29.201, 252}, {29.234, 250}, {29.267, 254}, {29.3, 264}, {29.333, 276}, {29.368, 289}, {29.401, 298}, {29.434, 307}, {29.467, 313}, {29.5, 312}, {29.534, 314}, {29.567, 307}, {29.601, 299}, {29.634, 289}, {29.667, 280}, {29.701, 271}, {29.734, 262}, {29.767, 254}, {29.8, 251}, {29.834, 246}, {29.868, 243}, {29.901, 236}, {29.934, 237}, {29.967, 232}, {30.0, 227}, {30.034, 224}, {30.068, 221}, {30.101, 218}, {30.134, 215}, {30.167, 208}, {30.201, 208}, {30.234, 206}, {30.267, 206}, {30.301, 204}, {30.334, 209}, {30.368, 215}, {30.401, 221}, {30.434, 231}, {30.467, 236}, {30.5, 241}, {30.535, 245}, {30.568, 251}, {30.601, 258}, {30.634, 265}, {30.667, 273}, {30.701, 277}, {30.735, 281}, {30.768, 287}, {30.801, 293}, {30.834, 298}, {30.868, 302}, {30.901, 307}, {30.934, 313}, {30.967, 317}, {31.0, 323}, {31.034, 322}, {31.067, 323}, {31.101, 328}, {31.134, 335}, {31.167, 340}, {31.201, 349}, {31.234, 348}, {31.267, 349}, {31.3, 349}, {31.334, 346}, {31.368, 342}, {31.401, 338}, {31.434, 332}, {31.467, 325}, {31.5, 322}, {31.534, 317}, {31.567, 324}, {31.601, 330}, {31.634, 340}, {31.667, 348}, {31.701, 359}, {31.734, 370}, {31.767, 379}, {31.8, 382}, {31.833, 381}, {31.868, 384}, {31.901, 383}, {31.934, 381}, {31.967, 378}, {32.0, 374}, {32.034, 372}, {32.068, 367}, {32.101, 362}, {32.134, 360}, {32.167, 361}, {32.201, 363}, {32.234, 364}, {32.267, 366}, {32.301, 368}, {32.334, 370}, {32.368, 366}, {32.401, 359}, {32.434, 353}, {32.467, 346}, {32.5, 333}, {32.535, 329}, {32.568, 320}, {32.601, 314}, {32.634, 308}, {32.667, 301}, {32.701, 295}, {32.734, 291}, {32.768, 284}, {32.801, 278}, {32.834, 275}, {32.868, 271}, {32.901, 270}, {32.934, 269}, {32.967, 272}, {33.0, 274}, {33.035, 276}, {33.068, 277}, {33.101, 277}, {33.134, 274}, {33.167, 273}, {33.201, 271}, {33.234, 268}, {33.267, 268}, {33.301, 262}, {33.334, 261}, {33.368, 261}, {33.401, 260}, {33.434, 262}, {33.467, 264}, {33.5, 264}, {33.535, 264}, {33.568, 262}, {33.601, 258}, {33.634, 252}, {33.667, 246}, {33.701, 238}, {33.734, 231}, {33.768, 222}, {33.801, 215}, {33.834, 211}, {33.868, 206}, {33.901, 203}, {33.934, 204}, {33.967, 203}, {34.0, 201}, {34.035, 196}, {34.068, 194}, {34.101, 190}, {34.134, 189}, {34.167, 181}, {34.201, 182}, {34.234, 182}, {34.268, 181}, {34.301, 184}, {34.334, 191}, {34.368, 200}, {34.401, 211}, {34.434, 223}, {34.467, 236}, {34.501, 248}, {34.535, 257}, {34.568, 261}, {34.601, 264}, {34.634, 263}, {34.667, 261}, {34.701, 259}, {34.735, 254}, {34.768, 253}, {34.801, 254}, {34.834, 260}, {34.868, 269}, {34.901, 279}, {34.934, 290}, {34.967, 300}, {35.0, 310}, {35.035, 320}, {35.068, 325}, {35.101, 328}, {35.134, 329}, {35.167, 328}, {35.201, 327}, {35.234, 325}, {35.268, 324}, {35.301, 324}, {35.334, 327}, {35.368, 331}, {35.401, 337}, {35.434, 343}, {35.467, 350}, {35.5, 355}, {35.534, 360}, {35.568, 362}, {35.601, 361}, {35.634, 360}, {35.667, 353}, {35.701, 346}, {35.734, 339}, {35.767, 331}, {35.801, 322}, {35.834, 317}, {35.868, 315}, {35.901, 317}, {35.934, 318}, {35.967, 319}, {36.0, 321}, {36.035, 324}, {36.068, 329}, {36.101, 328}, {36.134, 329}, {36.167, 332}, {36.201, 327}, {36.234, 323}, {36.268, 318}, {36.301, 309}, {36.334, 303}, {36.368, 295}, {36.401, 285}, {36.434, 277}, {36.468, 272}, {36.501, 269}, {36.535, 268}, {36.568, 272}, {36.601, 279}, {36.634, 293}, {36.667, 303}, {36.701, 314}, {36.734, 325}, {36.768, 335}, {36.801, 345}, {36.834, 346}, {36.868, 338}, {36.901, 326}, {36.934, 316}, {36.967, 305}, {37.001, 295}, {37.035, 286}, {37.068, 280}, {37.101, 279}, {37.134, 285}, {37.167, 291}, {37.201, 296}, {37.234, 302}, {37.268, 307}, {37.301, 308}, {37.334, 308}, {37.368, 307}, {37.401, 302}, {37.434, 304}, {37.467, 298}, {37.5, 292}, {37.535, 290}, {37.568, 290}, {37.601, 296}, {37.634, 301}, {37.667, 308}, {37.701, 313}, {37.734, 315}, {37.768, 316}, {37.801, 311}, {37.834, 305}, {37.868, 298}, {37.901, 290}, {37.934, 284}, {37.967, 278}, {38.0, 272}, {38.035, 269}, {38.068, 269}, {38.101, 267}, {38.134, 266}, {38.167, 265}, {38.201, 270}, {38.234, 277}, {38.268, 285}, {38.301, 294}, {38.334, 305}, {38.368, 316}, {38.401, 325}, {38.434, 330}, {38.467, 331}, {38.5, 328}, {38.535, 327}, {38.568, 318}, {38.601, 302}, {38.634, 296}, {38.667, 286}, {38.701, 287}, {38.735, 285}, {38.768, 293}, {38.801, 302}, {38.834, 311}, {38.868, 321}, {38.901, 332}, {38.934, 339}, {38.967, 345}, {39.001, 347}, {39.035, 344}, {39.068, 343}, {39.101, 337}, {39.134, 334}, {39.167, 332}, {39.201, 329}, {39.234, 331}, {39.268, 332}, {39.301, 334}, {39.334, 341}, {39.368, 350}, {39.401, 359}, {39.434, 365}, {39.467, 368}, {39.5, 372}, {39.534, 371}, {39.568, 368}, {39.601, 365}, {39.634, 360}, {39.667, 357}, {39.701, 357}, {39.734, 356}, {39.767, 357}, {39.801, 360}, {39.834, 361}, {39.868, 365}, {39.901, 361}, {39.934, 362}, {39.967, 355}, {40.0, 345}, {40.034, 333}, {40.068, 323}, {40.101, 311}, {40.134, 304}, {40.167, 296}, {40.201, 291}, {40.234, 285}, {40.268, 283}, {40.301, 284}, {40.334, 291}, {40.368, 292}, {40.401, 297}, {40.434, 302}, {40.468, 307}, {40.501, 312}, {40.535, 315}, {40.568, 317}, {40.601, 318}, {40.634, 316}, {40.667, 315}, {40.701, 308}, {40.735, 301}, {40.768, 296}, {40.801, 291}, {40.834, 291}, {40.868, 289}, {40.901, 287}, {40.935, 293}, {40.968, 299}, {41.001, 311}, {41.035, 322}, {41.068, 334}, {41.101, 345}, {41.134, 354}, {41.167, 355}, {41.201, 353}, {41.234, 349}, {41.268, 344}, {41.301, 336}, {41.334, 326}, {41.368, 318}, {41.401, 312}, {41.434, 311}, {41.467, 317}, {41.501, 323}, {41.535, 331}, {41.568, 338}, {41.601, 346}, {41.634, 351}, {41.667, 356}, {41.701, 352}, {41.734, 350}, {41.767, 344}, {41.801, 334}, {41.834, 324}, {41.868, 315}, {41.901, 307}, {41.934, 304}, {41.967, 301}, {42.001, 301}, {42.035, 306}, {42.068, 312}, {42.101, 315}, {42.134, 320}, {42.167, 323}, {42.201, 326}, {42.235, 329}, {42.268, 327}, {42.301, 326}, {42.334, 324}, {42.368, 317}, {42.401, 308}, {42.434, 302}, {42.468, 296}, {42.501, 296}, {42.535, 291}, {42.568, 292}, {42.601, 296}, {42.634, 303}, {42.668, 310}, {42.701, 317}, {42.735, 319}, {42.768, 324}, {42.801, 321}, {42.834, 320}, {42.868, 318}, {42.901, 316}, {42.934, 311}, {42.968, 307}, {43.001, 301}, {43.035, 297}, {43.068, 296}, {43.101, 297}, {43.134, 305}, {43.167, 310}, {43.201, 315}, {43.235, 321}, {43.268, 332}, {43.301, 335}, {43.334, 333}, {43.368, 332}, {43.401, 328}, {43.434, 321}, {43.467, 314}, {43.501, 308}, {43.535, 299}, {43.568, 293}, {43.601, 289}, {43.634, 289}, {43.667, 290}, {43.701, 293}, {43.734, 296}, {43.768, 297}, {43.801, 297}, {43.834, 295}, {43.868, 287}, {43.901, 280}, {43.934, 273}, {43.967, 267}, {44.001, 261}, {44.035, 254}, {44.068, 250}, {44.101, 246}, {44.134, 245}, {44.167, 244}, {44.201, 247}, {44.235, 256}, {44.268, 259}, {44.301, 269}, {44.334, 277}, {44.368, 284}, {44.401, 286}, {44.434, 283}, {44.468, 280}, {44.501, 277}, {44.535, 269}, {44.568, 266}, {44.601, 266}, {44.634, 265}, {44.667, 272}, {44.701, 280}, {44.735, 293}, {44.768, 304}, {44.801, 320}, {44.834, 331}, {44.868, 338}, {44.901, 344}, {44.934, 342}, {44.967, 336}, {45.001, 329}, {45.035, 323}, {45.068, 323}, {45.101, 326}, {45.134, 335}, {45.167, 344}, {45.201, 353}, {45.234, 360}, {45.267, 368}, {45.301, 374}, {45.334, 374}, {45.368, 373}, {45.401, 368}, {45.434, 362}, {45.467, 358}, {45.501, 358}, {45.535, 359}, {45.568, 362}, {45.601, 365}, {45.634, 367}, {45.667, 369}, {45.701, 369}, {45.735, 373}, {45.768, 375}, {45.801, 378}, {45.834, 382}, {45.868, 385}, {45.901, 388}, {45.934, 395}, {45.967, 395}, {46.0, 400}, {46.034, 403}, {46.068, 401}, {46.101, 399}, {46.134, 393}, {46.167, 388}, {46.201, 383}, {46.234, 379}, {46.268, 378}, {46.301, 379}, {46.334, 379}, {46.368, 378}, {46.401, 375}, {46.434, 367}, {46.467, 364}, {46.5, 359}, {46.535, 353}, {46.568, 348}, {46.601, 348}, {46.634, 347}, {46.667, 348}, {46.701, 349}, {46.734, 349}, {46.768, 349}, {46.801, 346}, {46.834, 341}, {46.868, 338}, {46.901, 328}, {46.934, 319}, {46.968, 310}, {47.001, 304}, {47.035, 299}, {47.068, 297}, {47.101, 294}, {47.134, 295}, {47.168, 298}, {47.201, 301}, {47.235, 306}, {47.268, 311}, {47.301, 317}, {47.334, 323}, {47.368, 329}, {47.402, 332}, {47.435, 330}, {47.468, 323}, {47.501, 319}, {47.535, 314}, {47.568, 312}, {47.601, 309}, {47.634, 315}, {47.668, 322}, {47.701, 332}, {47.735, 342}, {47.768, 352}, {47.801, 363}, {47.834, 372}, {47.868, 379}, {47.901, 382}, {47.934, 383}, {47.968, 384}, {48.001, 384}, {48.035, 381}, {48.068, 380}, {48.101, 378}, {48.134, 377}, {48.168, 376}, {48.201, 377}, {48.235, 376}, {48.268, 376}, {48.301, 378}, {48.334, 380}, {48.368, 384}, {48.402, 387}, {48.435, 389}, {48.468, 391}, {48.501, 393}, {48.535, 394}, {48.568, 394}, {48.601, 392}, {48.635, 391}, {48.668, 390}, {48.701, 390}, {48.735, 390}, {48.768, 389}, {48.801, 390}, {48.835, 392}, {48.868, 395}, {48.902, 398}, {48.935, 401}, {48.968, 403}, {49.001, 403}, {49.035, 400}, {49.068, 398}, {49.102, 395}, {49.135, 391}, {49.168, 392}, {49.201, 382}, {49.235, 378}, {49.268, 376}, {49.302, 374}, {49.335, 373}, {49.368, 372}, {49.402, 372}, {49.435, 373}, {49.468, 375}, {49.501, 378}, {49.535, 380}, {49.569, 382}, {49.602, 383}, {49.635, 380}, {49.668, 375}, {49.701, 368}, {49.735, 363}, {49.769, 358}, {49.802, 354}, {49.835, 348}, {49.868, 343}, {49.902, 343}, {49.935, 344}, {49.969, 344}, {50.002, 347}, {50.035, 355}, {50.069, 355}, {50.102, 360}, {50.135, 366}, {50.168, 370}, {50.201, 376}, {50.235, 380}, {50.269, 381}, {50.301, 378}, {50.335, 376}, {50.368, 371}, {50.402, 366}, {50.435, 360}, {50.468, 355}, {50.501, 353}, {50.535, 352}, {50.569, 350}, {50.602, 348}, {50.635, 345}, {50.668, 342}, {50.701, 340}, {50.735, 343}, {50.769, 343}, {50.802, 342}, {50.835, 346}, {50.868, 343}, {50.902, 345}, {50.935, 346}, {50.968, 344}, {51.001, 340}, {51.035, 335}, {51.069, 328}, {51.102, 322}, {51.135, 315}, {51.168, 309}, {51.201, 303}, {51.235, 298}, {51.269, 293}, {51.302, 287}, {51.335, 286}, {51.368, 290}, {51.402, 292}, {51.435, 297}, {51.468, 305}, {51.502, 311}, {51.535, 321}, {51.569, 328}, {51.602, 333}, {51.635, 337}, {51.668, 342}, {51.701, 337}, {51.735, 333}, {51.768, 328}, {51.802, 321}, {51.835, 314}, {51.868, 306}, {51.902, 302}, {51.935, 304}, {51.968, 311}, {52.001, 321}, {52.035, 328}, {52.069, 341}, {52.102, 349}, {52.135, 361}, {52.168, 373}, {52.201, 374}, {52.235, 375}, {52.268, 375}, {52.301, 373}, {52.335, 369}, {52.368, 363}, {52.402, 359}, {52.435, 353}, {52.468, 348}, {52.501, 343}, {52.535, 337}, {52.568, 336}, {52.602, 337}, {52.635, 337}, {52.668, 334}, {52.701, 331}, {52.735, 330}, {52.768, 327}, {52.802, 326}, {52.835, 320}, {52.868, 319}, {52.902, 321}, {52.935, 313}, {52.968, 310}, {53.002, 302}, {53.035, 293}, {53.069, 282}, {53.102, 275}, {53.135, 267}, {53.168, 258}, {53.201, 251}, {53.236, 246}, {53.269, 245}, {53.302, 248}, {53.335, 252}, {53.368, 262}, {53.402, 275}, {53.435, 285}, {53.468, 297}, {53.502, 306}, {53.535, 312}, {53.569, 319}, {53.602, 321}, {53.635, 323}, {53.668, 318}, {53.701, 315}, {53.735, 308}, {53.769, 305}, {53.802, 311}, {53.835, 312}, {53.868, 323}, {53.902, 334}, {53.935, 347}, {53.968, 359}, {54.001, 371}, {54.035, 379}, {54.069, 384}, {54.101, 385}, {54.135, 378}, {54.168, 369}, {54.201, 359}, {54.235, 350}, {54.268, 342}, {54.302, 337}, {54.335, 335}, {54.368, 335}, {54.402, 341}, {54.435, 346}, {54.468, 352}, {54.501, 360}, {54.535, 364}, {54.568, 368}, {54.601, 368}, {54.635, 365}, {54.668, 359}, {54.701, 351}, {54.735, 339}, {54.768, 330}, {54.802, 320}, {54.834, 309}, {54.868, 301}, {54.902, 297}, {54.935, 291}, {54.968, 291}, {55.001, 292}, {55.035, 299}, {55.069, 299}, {55.102, 304}, {55.135, 310}, {55.168, 314}, {55.201, 320}, {55.235, 325}, {55.268, 330}, {55.302, 332}, {55.335, 331}, {55.368, 331}, {55.402, 323}, {55.435, 319}, {55.468, 313}, {55.501, 313}, {55.535, 319}, {55.569, 324}, {55.602, 331}, {55.635, 338}, {55.668, 344}, {55.701, 350}, {55.735, 354}, {55.768, 354}, {55.802, 352}, {55.835, 349}, {55.868, 345}, {55.902, 342}, {55.935, 337}, {55.968, 332}, {56.001, 329}, {56.035, 328}, {56.068, 326}, {56.102, 325}, {56.135, 326}, {56.168, 328}, {56.201, 332}, {56.235, 333}, {56.268, 339}, {56.301, 336}, {56.335, 334}, {56.368, 331}, {56.402, 325}, {56.435, 316}, {56.468, 309}, {56.501, 298}, {56.535, 289}, {56.568, 282}, {56.602, 276}, {56.635, 275}, {56.668, 275}, {56.701, 277}, {56.735, 282}, {56.769, 286}, {56.802, 292}, {56.835, 295}, {56.868, 296}, {56.902, 293}, {56.935, 288}, {56.968, 282}, {57.001, 271}, {57.035, 265}, {57.069, 256}, {57.102, 247}, {57.135, 242}, {57.168, 239}, {57.201, 238}, {57.235, 240}, {57.269, 243}, {57.302, 247}, {57.335, 252}, {57.368, 258}, {57.402, 265}, {57.435, 271}, {57.469, 279}, {57.502, 285}, {57.535, 293}, {57.569, 298}, {57.602, 305}, {57.635, 309}, {57.668, 311}, {57.701, 310}, {57.735, 311}, {57.769, 309}, {57.802, 305}, {57.835, 301}, {57.868, 302}, {57.902, 312}, {57.935, 322}, {57.968, 335}, {58.001, 349}, {58.043, 363}, {58.069, 371}, {58.102, 372}, {58.135, 371}, {58.168, 368}, {58.201, 365}, {58.235, 361}, {58.268, 358}, {58.302, 360}, {58.335, 364}, {58.368, 374}, {58.402, 382}, {58.435, 389}, {58.468, 398}, {58.501, 402}, {58.535, 401}, {58.569, 396}, {58.602, 387}, {58.635, 383}, {58.668, 371}, {58.701, 362}, {58.744, 356}, {58.769, 353}, {58.802, 354}, {58.835, 352}, {58.868, 355}, {58.902, 354}, {58.935, 353}, {58.969, 349}, {59.007, 341}, {59.035, 332}, {59.069, 323}, {59.102, 316}, {59.135, 313}, {59.168, 309}, {59.201, 307}, {59.236, 306}, {59.269, 310}, {59.302, 310}, {59.335, 307}, {59.368, 302}, {59.402, 296}, {59.435, 288}, {59.468, 282}, {59.502, 276}, {59.535, 271}, {59.569, 268}, {59.602, 265}, {59.635, 262}, {59.668, 263}, {59.701, 265}, {59.735, 269}, {59.769, 274}, {59.802, 281}, {59.835, 277}, {59.868, 276}, {59.902, 273}, {59.935, 263}, {59.968, 255}, {60.001, 249}]}]
  out "FPS":i32=30
  out "time (s)":dbl[](array[numeric])=[0.0, 0.034, 0.067, 0.1, 0.133, 0.167, 0.201, 0.234, 0.267, 0.3, 0.333, 0.367, 0.401, 0.434, 0.467, 0.5, 0.534, 0.567, 0.601, 0.634, 0.667, 0.701, 0.734, 0.767, 0.8, 0.833, 0.867, 0.901, 0.934, 0.967, 1.0, 1.034, 1.067, 1.1, 1.134, 1.167, 1.201, 1.234, 1.267, 1.3, 1.333, 1.367, 1.401, 1.434, 1.467, 1.5, 1.534, 1.567, 1.6, 1.633, 1.666, 1.701, 1.734, 1.767, 1.8, 1.833, 1.867, 1.9, 1.933, 1.967, 2.0, 2.034, 2.067, 2.1, 2.133, 2.166, 2.201, 2.234, 2.267, 2.3, 2.333, 2.367, 2.4, 2.434, 2.467, 2.5, 2.534, 2.567, 2.6, 2.633, 2.666, 2.701, 2.734, 2.767, 2.8, 2.833, 2.867, 2.901, 2.934, 2.967, 3.0, 3.034, 3.067, 3.101, 3.134, 3.167, 3.201, 3.234, 3.267, 3.3, 3.333, 3.368, 3.401, 3.434, 3.467, 3.5, 3.534, 3.567, 3.6, 3.634, 3.667, 3.701, 3.734, 3.767, 3.8, 3.833, 3.868, 3.901, 3.934, 3.967, 4.0, 4.034, 4.068, 4.101, 4.134, 4.167, 4.201, 4.234, 4.267, 4.3, 4.333, 4.367, 4.4, 4.434, 4.467, 4.5, 4.534, 4.567, 4.6, 4.633, 4.667, 4.701, 4.734, 4.767, 4.8, 4.833, 4.867, 4.9, 4.933, 4.966, 5.0, 5.034, 5.067, 5.1, 5.133, 5.166, 5.2, 5.234, 5.267, 5.3, 5.333, 5.367, 5.4, 5.433, 5.467, 5.5, 5.534, 5.567, 5.6, 5.633, 5.666, 5.7, 5.733, 5.767, 5.8, 5.833, 5.867, 5.9, 5.933, 5.967, 6.0, 6.034, 6.067, 6.1, 6.133, 6.166, 6.2, 6.233, 6.266, 6.299, 6.333, 6.367, 6.4, 6.433, 6.467, 6.5, 6.534, 6.567, 6.6, 6.633, 6.666, 6.701, 6.734, 6.767, 6.8, 6.833, 6.867, 6.901, 6.934, 6.967, 7.0, 7.034, 7.067, 7.101, 7.134, 7.167, 7.201, 7.234, 7.267, 7.301, 7.334, 7.368, 7.401, 7.434, 7.467, 7.5, 7.534, 7.568, 7.601, 7.634, 7.667, 7.701, 7.734, 7.767, 7.801, 7.834, 7.868, 7.901, 7.934, 7.967, 8.0, 8.034, 8.068, 8.101, 8.134, 8.167, 8.201, 8.234, 8.268, 8.301, 8.334, 8.368, 8.401, 8.434, 8.467, 8.5, 8.534, 8.568, 8.601, 8.634, 8.667, 8.701, 8.734, 8.767, 8.8, 8.833, 8.867, 8.901, 8.934, 8.967, 9.0, 9.034, 9.067, 9.1, 9.133, 9.167, 9.201, 9.234, 9.267, 9.3, 9.333, 9.367, 9.4, 9.433, 9.467, 9.5, 9.534, 9.567, 9.6, 9.633, 9.666, 9.701, 9.734, 9.767, 9.8, 9.833, 9.867, 9.9, 9.934, 9.967, 10.0, 10.034, 10.067, 10.1, 10.133, 10.167, 10.201, 10.234, 10.267, 10.3, 10.333, 10.367, 10.4, 10.433, 10.467, 10.5, 10.534, 10.567, 10.6, 10.633, 10.667, 10.701, 10.734, 10.767, 10.8, 10.833, 10.867, 10.901, 10.934, 10.967, 11.0, 11.034, 11.067, 11.101, 11.134, 11.167, 11.201, 11.234, 11.267, 11.3, 11.333, 11.368, 11.401, 11.434, 11.467, 11.5, 11.535, 11.568, 11.601, 11.634, 11.667, 11.701, 11.734, 11.768, 11.8, 11.834, 11.868, 11.901, 11.934, 11.967, 12.0, 12.034, 12.067, 12.101, 12.134, 12.167, 12.201, 12.234, 12.267, 12.3, 12.334, 12.368, 12.401, 12.434, 12.467, 12.5, 12.535, 12.568, 12.601, 12.634, 12.667, 12.701, 12.735, 12.768, 12.801, 12.834, 12.868, 12.901, 12.934, 12.967, 13.0, 13.035, 13.068, 13.101, 13.134, 13.167, 13.201, 13.234, 13.268, 13.301, 13.334, 13.368, 13.401, 13.434, 13.467, 13.5, 13.534, 13.567, 13.6, 13.634, 13.667, 13.701, 13.734, 13.767, 13.8, 13.833, 13.867, 13.901, 13.934, 13.967, 14.0, 14.034, 14.067, 14.1, 14.133, 14.166, 14.201, 14.234, 14.267, 14.3, 14.333, 14.367, 14.4, 14.433, 14.467, 14.5, 14.534, 14.567, 14.6, 14.633, 14.666, 14.7, 14.734, 14.767, 14.8, 14.833, 14.867, 14.9, 14.934, 14.967, 15.0, 15.034, 15.067, 15.1, 15.133, 15.167, 15.201, 15.234, 15.267, 15.3, 15.334, 15.368, 15.401, 15.434, 15.467, 15.5, 15.535, 15.568, 15.601, 15.634, 15.667, 15.701, 15.735, 15.768, 15.801, 15.834, 15.868, 15.901, 15.934, 15.967, 16.001, 16.035, 16.068, 16.101, 16.134, 16.167, 16.201, 16.234, 16.267, 16.3, 16.334, 16.368, 16.401, 16.434, 16.467, 16.5, 16.534, 16.568, 16.601, 16.634, 16.667, 16.701, 16.734, 16.768, 16.801, 16.834, 16.868, 16.901, 16.934, 16.968, 17.001, 17.035, 17.068, 17.101, 17.134, 17.167, 17.201, 17.235, 17.268, 17.301, 17.334, 17.368, 17.401, 17.435, 17.468, 17.501, 17.535, 17.568, 17.601, 17.634, 17.667, 17.701, 17.735, 17.768, 17.801, 17.834, 17.868, 17.901, 17.934, 17.968, 18.001, 18.035, 18.068, 18.101, 18.134, 18.167, 18.201, 18.234, 18.267, 18.301, 18.334, 18.368, 18.401, 18.434, 18.467, 18.5, 18.534, 18.568, 18.601, 18.634, 18.667, 18.701, 18.734, 18.768, 18.801, 18.834, 18.868, 18.901, 18.935, 18.968, 19.001, 19.035, 19.068, 19.101, 19.134, 19.167, 19.201, 19.235, 19.268, 19.301, 19.334, 19.368, 19.401, 19.435, 19.468, 19.501, 19.535, 19.568, 19.601, 19.634, 19.667, 19.701, 19.735, 19.768, 19.801, 19.834, 19.868, 19.901, 19.934, 19.967, 20.001, 20.035, 20.068, 20.101, 20.134, 20.167, 20.201, 20.235, 20.268, 20.301, 20.334, 20.368, 20.401, 20.434, 20.468, 20.501, 20.535, 20.568, 20.601, 20.634, 20.667, 20.701, 20.735, 20.768, 20.801, 20.834, 20.868, 20.901, 20.934, 20.968, 21.001, 21.035, 21.068, 21.101, 21.134, 21.167, 21.201, 21.235, 21.268, 21.301, 21.334, 21.368, 21.401, 21.434, 21.468, 21.501, 21.535, 21.568, 21.601, 21.634, 21.667, 21.701, 21.734, 21.768, 21.801, 21.834, 21.868, 21.901, 21.934, 21.967, 22.0, 22.034, 22.068, 22.101, 22.134, 22.167, 22.201, 22.234, 22.267, 22.3, 22.333, 22.368, 22.401, 22.434, 22.467, 22.5, 22.534, 22.567, 22.601, 22.634, 22.667, 22.701, 22.734, 22.767, 22.8, 22.834, 22.868, 22.901, 22.934, 22.967, 23.0, 23.034, 23.067, 23.1, 23.134, 23.167, 23.201, 23.234, 23.267, 23.3, 23.334, 23.368, 23.401, 23.434, 23.467, 23.5, 23.535, 23.568, 23.601, 23.634, 23.667, 23.701, 23.735, 23.768, 23.801, 23.834, 23.868, 23.901, 23.934, 23.968, 24.001, 24.035, 24.068, 24.101, 24.134, 24.168, 24.201, 24.235, 24.268, 24.301, 24.334, 24.368, 24.402, 24.435, 24.468, 24.501, 24.535, 24.568, 24.601, 24.634, 24.668, 24.701, 24.735, 24.768, 24.801, 24.834, 24.868, 24.901, 24.935, 24.968, 25.001, 25.035, 25.068, 25.101, 25.134, 25.168, 25.201, 25.235, 25.268, 25.301, 25.334, 25.368, 25.401, 25.434, 25.468, 25.501, 25.535, 25.568, 25.601, 25.634, 25.667, 25.701, 25.735, 25.768, 25.801, 25.834, 25.868, 25.901, 25.934, 25.967, 26.001, 26.035, 26.068, 26.101, 26.134, 26.167, 26.201, 26.234, 26.268, 26.301, 26.334, 26.368, 26.401, 26.434, 26.467, 26.5, 26.535, 26.568, 26.601, 26.634, 26.667, 26.701, 26.734, 26.767, 26.801, 26.834, 26.868, 26.901, 26.934, 26.967, 27.0, 27.035, 27.068, 27.101, 27.134, 27.167, 27.201, 27.234, 27.267, 27.3, 27.334, 27.368, 27.401, 27.434, 27.467, 27.5, 27.534, 27.567, 27.6, 27.634, 27.667, 27.701, 27.734, 27.767, 27.8, 27.833, 27.868, 27.901, 27.934, 27.967, 28.0, 28.034, 28.067, 28.1, 28.134, 28.167, 28.201, 28.234, 28.267, 28.3, 28.333, 28.368, 28.401, 28.434, 28.467, 28.5, 28.534, 28.567, 28.6, 28.634, 28.667, 28.701, 28.734, 28.767, 28.801, 28.834, 28.868, 28.901, 28.934, 28.967, 29.0, 29.034, 29.068, 29.101, 29.134, 29.167, 29.201, 29.234, 29.267, 29.3, 29.333, 29.368, 29.401, 29.434, 29.467, 29.5, 29.534, 29.567, 29.601, 29.634, 29.667, 29.701, 29.734, 29.767, 29.8, 29.834, 29.868, 29.901, 29.934, 29.967, 30.0, 30.034, 30.068, 30.101, 30.134, 30.167, 30.201, 30.234, 30.267, 30.301, 30.334, 30.368, 30.401, 30.434, 30.467, 30.5, 30.535, 30.568, 30.601, 30.634, 30.667, 30.701, 30.735, 30.768, 30.801, 30.834, 30.868, 30.901, 30.934, 30.967, 31.0, 31.034, 31.067, 31.101, 31.134, 31.167, 31.201, 31.234, 31.267, 31.3, 31.334, 31.368, 31.401, 31.434, 31.467, 31.5, 31.534, 31.567, 31.601, 31.634, 31.667, 31.701, 31.734, 31.767, 31.8, 31.833, 31.868, 31.901, 31.934, 31.967, 32.0, 32.034, 32.068, 32.101, 32.134, 32.167, 32.201, 32.234, 32.267, 32.301, 32.334, 32.368, 32.401, 32.434, 32.467, 32.5, 32.535, 32.568, 32.601, 32.634, 32.667, 32.701, 32.734, 32.768, 32.801, 32.834, 32.868, 32.901, 32.934, 32.967, 33.0, 33.035, 33.068, 33.101, 33.134, 33.167, 33.201, 33.234, 33.267, 33.301, 33.334, 33.368, 33.401, 33.434, 33.467, 33.5, 33.535, 33.568, 33.601, 33.634, 33.667, 33.701, 33.734, 33.768, 33.801, 33.834, 33.868, 33.901, 33.934, 33.967, 34.0, 34.035, 34.068, 34.101, 34.134, 34.167, 34.201, 34.234, 34.268, 34.301, 34.334, 34.368, 34.401, 34.434, 34.467, 34.501, 34.535, 34.568, 34.601, 34.634, 34.667, 34.701, 34.735, 34.768, 34.801, 34.834, 34.868, 34.901, 34.934, 34.967, 35.0, 35.035, 35.068, 35.101, 35.134, 35.167, 35.201, 35.234, 35.268, 35.301, 35.334, 35.368, 35.401, 35.434, 35.467, 35.5, 35.534, 35.568, 35.601, 35.634, 35.667, 35.701, 35.734, 35.767, 35.801, 35.834, 35.868, 35.901, 35.934, 35.967, 36.0, 36.035, 36.068, 36.101, 36.134, 36.167, 36.201, 36.234, 36.268, 36.301, 36.334, 36.368, 36.401, 36.434, 36.468, 36.501, 36.535, 36.568, 36.601, 36.634, 36.667, 36.701, 36.734, 36.768, 36.801, 36.834, 36.868, 36.901, 36.934, 36.967, 37.001, 37.035, 37.068, 37.101, 37.134, 37.167, 37.201, 37.234, 37.268, 37.301, 37.334, 37.368, 37.401, 37.434, 37.467, 37.5, 37.535, 37.568, 37.601, 37.634, 37.667, 37.701, 37.734, 37.768, 37.801, 37.834, 37.868, 37.901, 37.934, 37.967, 38.0, 38.035, 38.068, 38.101, 38.134, 38.167, 38.201, 38.234, 38.268, 38.301, 38.334, 38.368, 38.401, 38.434, 38.467, 38.5, 38.535, 38.568, 38.601, 38.634, 38.667, 38.701, 38.735, 38.768, 38.801, 38.834, 38.868, 38.901, 38.934, 38.967, 39.001, 39.035, 39.068, 39.101, 39.134, 39.167, 39.201, 39.234, 39.268, 39.301, 39.334, 39.368, 39.401, 39.434, 39.467, 39.5, 39.534, 39.568, 39.601, 39.634, 39.667, 39.701, 39.734, 39.767, 39.801, 39.834, 39.868, 39.901, 39.934, 39.967, 40.0, 40.034, 40.068, 40.101, 40.134, 40.167, 40.201, 40.234, 40.268, 40.301, 40.334, 40.368, 40.401, 40.434, 40.468, 40.501, 40.535, 40.568, 40.601, 40.634, 40.667, 40.701, 40.735, 40.768, 40.801, 40.834, 40.868, 40.901, 40.935, 40.968, 41.001, 41.035, 41.068, 41.101, 41.134, 41.167, 41.201, 41.234, 41.268, 41.301, 41.334, 41.368, 41.401, 41.434, 41.467, 41.501, 41.535, 41.568, 41.601, 41.634, 41.667, 41.701, 41.734, 41.767, 41.801, 41.834, 41.868, 41.901, 41.934, 41.967, 42.001, 42.035, 42.068, 42.101, 42.134, 42.167, 42.201, 42.235, 42.268, 42.301, 42.334, 42.368, 42.401, 42.434, 42.468, 42.501, 42.535, 42.568, 42.601, 42.634, 42.668, 42.701, 42.735, 42.768, 42.801, 42.834, 42.868, 42.901, 42.934, 42.968, 43.001, 43.035, 43.068, 43.101, 43.134, 43.167, 43.201, 43.235, 43.268, 43.301, 43.334, 43.368, 43.401, 43.434, 43.467, 43.501, 43.535, 43.568, 43.601, 43.634, 43.667, 43.701, 43.734, 43.768, 43.801, 43.834, 43.868, 43.901, 43.934, 43.967, 44.001, 44.035, 44.068, 44.101, 44.134, 44.167, 44.201, 44.235, 44.268, 44.301, 44.334, 44.368, 44.401, 44.434, 44.468, 44.501, 44.535, 44.568, 44.601, 44.634, 44.667, 44.701, 44.735, 44.768, 44.801, 44.834, 44.868, 44.901, 44.934, 44.967, 45.001, 45.035, 45.068, 45.101, 45.134, 45.167, 45.201, 45.234, 45.267, 45.301, 45.334, 45.368, 45.401, 45.434, 45.467, 45.501, 45.535, 45.568, 45.601, 45.634, 45.667, 45.701, 45.735, 45.768, 45.801, 45.834, 45.868, 45.901, 45.934, 45.967, 46.0, 46.034, 46.068, 46.101, 46.134, 46.167, 46.201, 46.234, 46.268, 46.301, 46.334, 46.368, 46.401, 46.434, 46.467, 46.5, 46.535, 46.568, 46.601, 46.634, 46.667, 46.701, 46.734, 46.768, 46.801, 46.834, 46.868, 46.901, 46.934, 46.968, 47.001, 47.035, 47.068, 47.101, 47.134, 47.168, 47.201, 47.235, 47.268, 47.301, 47.334, 47.368, 47.402, 47.435, 47.468, 47.501, 47.535, 47.568, 47.601, 47.634, 47.668, 47.701, 47.735, 47.768, 47.801, 47.834, 47.868, 47.901, 47.934, 47.968, 48.001, 48.035, 48.068, 48.101, 48.134, 48.168, 48.201, 48.235, 48.268, 48.301, 48.334, 48.368, 48.402, 48.435, 48.468, 48.501, 48.535, 48.568, 48.601, 48.635, 48.668, 48.701, 48.735, 48.768, 48.801, 48.835, 48.868, 48.902, 48.935, 48.968, 49.001, 49.035, 49.068, 49.102, 49.135, 49.168, 49.201, 49.235, 49.268, 49.302, 49.335, 49.368, 49.402, 49.435, 49.468, 49.501, 49.535, 49.569, 49.602, 49.635, 49.668, 49.701, 49.735, 49.769, 49.802, 49.835, 49.868, 49.902, 49.935, 49.969, 50.002, 50.035, 50.069, 50.102, 50.135, 50.168, 50.201, 50.235, 50.269, 50.301, 50.335, 50.368, 50.402, 50.435, 50.468, 50.501, 50.535, 50.569, 50.602, 50.635, 50.668, 50.701, 50.735, 50.769, 50.802, 50.835, 50.868, 50.902, 50.935, 50.968, 51.001, 51.035, 51.069, 51.102, 51.135, 51.168, 51.201, 51.235, 51.269, 51.302, 51.335, 51.368, 51.402, 51.435, 51.468, 51.502, 51.535, 51.569, 51.602, 51.635, 51.668, 51.701, 51.735, 51.768, 51.802, 51.835, 51.868, 51.902, 51.935, 51.968, 52.001, 52.035, 52.069, 52.102, 52.135, 52.168, 52.201, 52.235, 52.268, 52.301, 52.335, 52.368, 52.402, 52.435, 52.468, 52.501, 52.535, 52.568, 52.602, 52.635, 52.668, 52.701, 52.735, 52.768, 52.802, 52.835, 52.868, 52.902, 52.935, 52.968, 53.002, 53.035, 53.069, 53.102, 53.135, 53.168, 53.201, 53.236, 53.269, 53.302, 53.335, 53.368, 53.402, 53.435, 53.468, 53.502, 53.535, 53.569, 53.602, 53.635, 53.668, 53.701, 53.735, 53.769, 53.802, 53.835, 53.868, 53.902, 53.935, 53.968, 54.001, 54.035, 54.069, 54.101, 54.135, 54.168, 54.201, 54.235, 54.268, 54.302, 54.335, 54.368, 54.402, 54.435, 54.468, 54.501, 54.535, 54.568, 54.601, 54.635, 54.668, 54.701, 54.735, 54.768, 54.802, 54.834, 54.868, 54.902, 54.935, 54.968, 55.001, 55.035, 55.069, 55.102, 55.135, 55.168, 55.201, 55.235, 55.268, 55.302, 55.335, 55.368, 55.402, 55.435, 55.468, 55.501, 55.535, 55.569, 55.602, 55.635, 55.668, 55.701, 55.735, 55.768, 55.802, 55.835, 55.868, 55.902, 55.935, 55.968, 56.001, 56.035, 56.068, 56.102, 56.135, 56.168, 56.201, 56.235, 56.268, 56.301, 56.335, 56.368, 56.402, 56.435, 56.468, 56.501, 56.535, 56.568, 56.602, 56.635, 56.668, 56.701, 56.735, 56.769, 56.802, 56.835, 56.868, 56.902, 56.935, 56.968, 57.001, 57.035, 57.069, 57.102, 57.135, 57.168, 57.201, 57.235, 57.269, 57.302, 57.335, 57.368, 57.402, 57.435, 57.469, 57.502, 57.535, 57.569, 57.602, 57.635, 57.668, 57.701, 57.735, 57.769, 57.802, 57.835, 57.868, 57.902, 57.935, 57.968, 58.001, 58.043, 58.069, 58.102, 58.135, 58.168, 58.201, 58.235, 58.268, 58.302, 58.335, 58.368, 58.402, 58.435, 58.468, 58.501, 58.535, 58.569, 58.602, 58.635, 58.668, 58.701, 58.744, 58.769, 58.802, 58.835, 58.868, 58.902, 58.935, 58.969, 59.007, 59.035, 59.069, 59.102, 59.135, 59.168, 59.201, 59.236, 59.269, 59.302, 59.335, 59.368, 59.402, 59.435, 59.468, 59.502, 59.535, 59.569, 59.602, 59.635, 59.668, 59.701, 59.735, 59.769, 59.802, 59.835, 59.868, 59.902, 59.935, 59.968, 60.001] format="%.3f"
  in  "Origin":cluster{"X":i32, "Y":i32}
  out "Y position vs time":cluster{dbl[], i32[]}(graph)
  out "X position vs time":cluster{dbl[], i32[]}(graph)
  in  "Pixel intensity\nthreshold":i32=55
  in  "Row min":i32=10
  in  "Row max":i32=470
  in  "Column min":i32=10
  in  "Column max":i32=630
  out "X positions\ncamera 1\n(image \ncoordinates)":i32[](array[numeric])=[251, 257, 266, 275, 283, 294, 308, 321, 332, 340, 346, 349, 351, 351, 350, 349, 350, 351, 352, 351, 351, 351, 350, 346, 343, 337, 331, 326, 322, 317, 314, 309, 304, 301, 298, 295, 291, 287, 282, 276, 269, 262, 258, 255, 252, 247, 244, 241, 238, 235, 232, 229, 227, 225, 222, 221, 220, 220, 220, 218, 219, 219, 217, 215, 216, 217, 220, 227, 238, 250, 261, 274, 283, 288, 294, 297, 297, 299, 302, 306, 313, 321, 330, 339, 348, 355, 364, 372, 380, 388, 395, 404, 412, 419, 427, 433, 441, 447, 453, 459, 463, 468, 472, 477, 483, 490, 496, 505, 512, 516, 521, 524, 524, 522, 521, 518, 513, 509, 504, 499, 495, 489, 482, 478, 476, 478, 483, 488, 493, 498, 500, 501, 499, 493, 485, 476, 465, 455, 443, 430, 418, 408, 399, 390, 379, 368, 360, 351, 342, 331, 321, 313, 305, 297, 290, 282, 275, 269, 262, 256, 249, 242, 238, 232, 228, 223, 221, 217, 212, 207, 200, 194, 191, 187, 183, 178, 173, 167, 161, 155, 149, 142, 136, 131, 127, 123, 121, 121, 120, 122, 124, 128, 135, 144, 155, 166, 177, 189, 202, 218, 233, 246, 255, 259, 259, 257, 254, 255, 261, 273, 290, 308, 325, 338, 350, 358, 367, 377, 386, 397, 407, 418, 428, 438, 449, 459, 467, 474, 481, 487, 492, 499, 506, 511, 515, 522, 530, 538, 540, 540, 538, 532, 521, 506, 493, 480, 469, 458, 447, 437, 425, 414, 403, 390, 378, 366, 356, 345, 333, 319, 309, 304, 300, 294, 285, 274, 263, 252, 242, 232, 220, 211, 200, 192, 185, 176, 168, 162, 157, 149, 142, 137, 135, 136, 140, 143, 144, 145, 146, 146, 145, 138, 133, 139, 146, 149, 149, 147, 147, 146, 144, 140, 140, 144, 150, 154, 157, 155, 156, 157, 157, 159, 160, 162, 166, 171, 178, 188, 198, 207, 213, 216, 219, 221, 226, 232, 240, 250, 259, 268, 275, 281, 288, 296, 308, 319, 331, 343, 353, 362, 372, 381, 392, 401, 409, 415, 420, 427, 436, 442, 449, 459, 468, 477, 487, 496, 502, 507, 511, 515, 523, 532, 540, 549, 556, 561, 562, 561, 558, 552, 546, 538, 528, 520, 513, 507, 500, 494, 489, 486, 484, 483, 480, 477, 476, 475, 473, 469, 463, 457, 450, 440, 429, 418, 409, 403, 401, 400, 400, 399, 395, 390, 383, 375, 364, 354, 346, 337, 327, 316, 307, 300, 293, 285, 279, 276, 273, 267, 261, 256, 251, 245, 239, 233, 224, 215, 207, 200, 193, 185, 177, 171, 164, 157, 152, 148, 142, 137, 134, 132, 130, 128, 126, 128, 130, 131, 134, 138, 143, 147, 152, 159, 169, 180, 194, 207, 220, 233, 247, 264, 282, 298, 314, 331, 346, 359, 371, 382, 394, 406, 416, 427, 438, 443, 444, 443, 435, 424, 412, 397, 382, 369, 358, 348, 338, 324, 311, 298, 286, 275, 265, 258, 252, 251, 254, 262, 274, 289, 303, 318, 331, 339, 345, 349, 350, 351, 353, 356, 358, 358, 358, 359, 361, 365, 370, 377, 388, 401, 413, 423, 433, 441, 446, 453, 457, 462, 467, 472, 477, 479, 481, 481, 482, 481, 477, 473, 466, 458, 449, 436, 419, 402, 383, 366, 350, 334, 321, 308, 295, 285, 274, 268, 264, 264, 267, 275, 281, 287, 292, 296, 301, 309, 318, 327, 339, 354, 369, 381, 393, 403, 411, 417, 424, 430, 438, 449, 461, 474, 484, 489, 489, 483, 472, 460, 447, 433, 418, 401, 384, 371, 364, 362, 357, 353, 350, 349, 348, 347, 347, 347, 346, 343, 341, 339, 336, 334, 331, 325, 322, 322, 321, 322, 325, 327, 331, 333, 335, 336, 336, 336, 338, 338, 335, 334, 335, 335, 336, 340, 344, 346, 345, 346, 346, 345, 345, 345, 349, 356, 363, 367, 372, 375, 376, 377, 381, 388, 392, 397, 403, 408, 409, 409, 407, 404, 400, 393, 381, 370, 359, 349, 339, 329, 321, 311, 303, 296, 290, 284, 279, 275, 270, 265, 259, 254, 250, 245, 240, 240, 238, 233, 229, 225, 223, 220, 218, 216, 212, 207, 204, 199, 194, 191, 188, 186, 185, 188, 196, 205, 217, 230, 242, 257, 270, 284, 299, 314, 328, 341, 351, 357, 359, 361, 364, 366, 369, 371, 373, 376, 380, 386, 393, 400, 407, 413, 418, 420, 424, 425, 425, 426, 426, 425, 426, 425, 423, 419, 415, 410, 404, 398, 391, 384, 380, 379, 379, 377, 375, 372, 367, 363, 358, 354, 349, 344, 338, 333, 331, 329, 325, 322, 318, 316, 315, 314, 313, 311, 310, 307, 303, 299, 295, 291, 286, 283, 279, 275, 269, 265, 263, 261, 258, 255, 254, 252, 251, 247, 242, 239, 237, 235, 232, 228, 223, 219, 215, 211, 207, 205, 202, 198, 195, 190, 185, 181, 176, 172, 169, 164, 158, 154, 151, 148, 144, 141, 137, 134, 132, 131, 130, 130, 129, 127, 123, 120, 117, 112, 108, 104, 99, 94, 90, 88, 85, 82, 79, 78, 78, 77, 76, 76, 78, 78, 77, 74, 74, 74, 74, 74, 75, 75, 74, 74, 74, 74, 76, 79, 84, 91, 99, 108, 113, 117, 122, 126, 129, 133, 135, 136, 134, 131, 129, 127, 124, 119, 114, 109, 102, 95, 90, 84, 76, 72, 73, 71, 69, 67, 66, 64, 64, 66, 68, 70, 72, 76, 78, 80, 82, 87, 89, 93, 97, 98, 99, 100, 103, 109, 116, 123, 129, 134, 138, 142, 147, 153, 158, 165, 172, 178, 182, 185, 186, 186, 183, 177, 170, 164, 158, 151, 142, 134, 128, 125, 121, 114, 108, 105, 103, 101, 99, 97, 95, 92, 88, 85, 82, 81, 79, 77, 75, 74, 72, 71, 71, 71, 74, 80, 84, 90, 96, 101, 107, 111, 115, 121, 126, 131, 136, 143, 149, 154, 157, 160, 162, 163, 164, 165, 166, 167, 168, 169, 167, 163, 158, 152, 147, 140, 133, 126, 122, 120, 116, 113, 110, 108, 105, 102, 101, 100, 97, 95, 93, 90, 89, 85, 82, 82, 81, 79, 79, 81, 83, 86, 89, 93, 96, 97, 98, 100, 99, 100, 104, 109, 115, 122, 130, 137, 139, 140, 142, 148, 153, 162, 172, 180, 186, 188, 187, 184, 180, 176, 171, 164, 158, 152, 147, 142, 140, 141, 143, 145, 145, 144, 143, 138, 131, 123, 116, 111, 105, 100, 98, 96, 95, 95, 95, 96, 95, 93, 94, 95, 95, 94, 91, 91, 90, 88, 85, 83, 82, 84, 87, 93, 101, 108, 115, 121, 126, 129, 133, 135, 135, 136, 137, 137, 133, 132, 132, 131, 130, 131, 133, 133, 133, 132, 130, 129, 129, 129, 129, 126, 122, 118, 114, 109, 102, 96, 94, 92, 91, 91, 90, 89, 86, 81, 77, 73, 68, 64, 59, 56, 54, 54, 53, 51, 51, 52, 53, 55, 56, 58, 61, 64, 65, 68, 72, 77, 80, 84, 88, 93, 96, 97, 97, 100, 103, 106, 110, 115, 124, 131, 136, 139, 141, 141, 143, 145, 149, 153, 156, 156, 155, 153, 151, 147, 141, 133, 126, 121, 119, 119, 116, 112, 109, 106, 102, 96, 92, 88, 83, 79, 75, 70, 68, 64, 60, 60, 63, 64, 66, 69, 74, 79, 82, 85, 87, 90, 92, 96, 100, 104, 109, 114, 120, 126, 131, 134, 138, 141, 144, 145, 146, 147, 146, 144, 141, 139, 138, 137, 135, 134, 132, 131, 130, 128, 125, 122, 120, 117, 113, 109, 107, 105, 104, 102, 98, 95, 93, 91, 90, 88, 86, 85, 83, 81, 80, 79, 79, 81, 84, 88, 93, 97, 103, 109, 115, 121, 125, 129, 131, 132, 132, 133, 136, 138, 138, 139, 144, 147, 150, 152, 152, 153, 152, 151, 149, 146, 144, 139, 134, 130, 125, 120, 115, 110, 104, 100, 97, 93, 90, 88, 85, 83, 80, 78, 77, 76, 74, 73, 75, 75, 74, 73, 74, 74, 74, 74, 74, 76, 76, 75, 76, 77, 78, 82, 87, 93, 100, 108, 114, 118, 121, 122, 122, 122, 121, 119, 115, 113, 112, 113, 116, 119, 121, 121, 118, 114, 108, 102, 98, 94, 90, 85, 78, 70, 65, 62, 61, 62, 63, 65, 68, 73, 80, 88, 94, 100, 106, 111, 117, 122, 128, 135, 140, 141, 138, 134, 128, 123, 121, 118, 114, 109, 105, 101, 98, 95, 91, 88, 85, 81, 81, 79, 77, 75, 71, 69, 70, 71, 71, 72, 75, 77, 79, 84, 90, 96, 101, 104, 107, 110, 110, 111, 113, 117, 121, 126, 131, 135, 140, 145, 148, 149, 149, 150, 154, 157, 161, 165, 170, 174, 178, 182, 186, 190, 192, 194, 197, 200, 204, 207, 209, 212, 216, 220, 226, 232, 238, 245, 253, 259, 265, 270, 273, 278, 284, 290, 296, 303, 312, 320, 329, 337, 345, 354, 362, 370, 379, 387, 396, 403, 411, 420, 427, 433, 439, 442, 446, 449, 452, 456, 460, 465, 471, 477, 484, 489, 494, 498, 499, 498, 496, 492, 486, 480, 474, 469, 466, 460, 453, 446, 441, 436, 430, 423, 415, 409, 403, 396, 390, 385, 378, 372, 368, 365, 364, 362, 359, 357, 354, 352, 349, 346, 344, 343, 341, 339, 337, 334, 331, 328, 326, 324, 322, 321, 321, 320, 319, 320, 321, 320, 320, 319, 319, 318, 318, 319, 319, 320, 321, 321, 320, 318, 314, 309, 302, 297, 294, 290, 284, 280, 275, 270, 267, 262, 258, 256, 256, 256, 254, 251, 249, 246, 242, 239, 237, 238, 241, 245, 250, 256, 263, 271, 276, 282, 290, 297, 303, 309, 314, 319, 323, 326, 328, 329, 329, 328, 327, 326, 324, 321, 317, 310, 303, 299, 295, 294, 294, 292, 290, 288, 287, 285, 282, 277, 271, 265, 260, 257, 255, 253, 250, 248, 245, 244, 243, 240, 237, 234, 230, 226, 222, 218, 214, 210, 208, 206, 202, 199, 196, 193, 190, 189, 189, 188, 187, 188, 192, 194, 197, 201, 207, 213, 221, 228, 235, 242, 247, 251, 252, 251, 251, 250, 250, 253, 255, 257, 258, 257, 256, 253, 251, 247, 242, 236, 230, 223, 216, 208, 202, 198, 192, 187, 184, 181, 178, 176, 175, 173, 170, 166, 161, 156, 151, 148, 145, 143, 143, 145, 147, 150, 156, 163, 170, 177, 185, 190, 195, 201, 205, 211, 216, 219, 222, 224, 227, 231, 236, 241, 247, 254, 260, 265, 269, 273, 277, 278, 278, 277, 274, 272, 270, 265, 258, 251, 247, 242, 237, 232, 228, 226, 226, 227, 230, 237, 245, 252, 259, 265, 272, 277, 281, 284, 289, 294, 297, 303, 309, 314, 320, 325, 330, 338, 346, 351, 354, 353, 349, 346, 340, 332, 326, 318, 309, 301, 292, 284, 277, 271, 264, 260, 258, 255, 251, 245, 239, 234, 229, 223, 217, 212, 211, 209, 208, 207, 205, 203, 200, 198, 197, 196, 195]
  out "Y positions camera 1 \n(image \ncoordinates)":i32[](array[numeric])=[275, 266, 249, 235, 224, 220, 209, 200, 202, 200, 192, 199, 202, 211, 212, 223, 227, 232, 235, 236, 233, 227, 216, 214, 201, 197, 189, 192, 194, 202, 211, 225, 241, 255, 267, 274, 279, 279, 277, 269, 267, 259, 252, 244, 240, 240, 238, 237, 239, 243, 251, 261, 273, 281, 291, 295, 294, 284, 274, 264, 247, 235, 225, 214, 206, 204, 204, 199, 201, 199, 198, 193, 187, 181, 169, 158, 149, 136, 125, 121, 112, 111, 115, 117, 118, 128, 127, 130, 131, 130, 133, 125, 119, 118, 113, 110, 103, 102, 105, 100, 100, 102, 104, 101, 108, 112, 114, 120, 127, 136, 148, 154, 168, 177, 187, 198, 209, 220, 231, 245, 258, 272, 289, 307, 324, 339, 353, 368, 382, 395, 406, 415, 420, 424, 422, 419, 414, 409, 403, 401, 397, 391, 391, 393, 398, 407, 413, 417, 420, 419, 418, 411, 405, 398, 391, 382, 377, 375, 371, 370, 369, 370, 369, 371, 374, 377, 381, 383, 388, 391, 395, 396, 391, 386, 379, 369, 361, 350, 343, 338, 336, 338, 342, 347, 354, 361, 368, 371, 370, 365, 358, 342, 330, 318, 310, 305, 304, 304, 307, 310, 317, 321, 326, 327, 326, 323, 316, 306, 302, 303, 311, 321, 337, 352, 363, 370, 366, 356, 343, 330, 321, 314, 313, 314, 315, 316, 318, 319, 318, 315, 311, 303, 301, 294, 296, 301, 308, 316, 324, 327, 325, 323, 317, 309, 300, 295, 291, 292, 293, 293, 293, 294, 294, 298, 297, 307, 307, 311, 318, 319, 315, 316, 308, 305, 304, 305, 306, 307, 309, 309, 309, 306, 305, 304, 303, 304, 306, 306, 304, 301, 298, 294, 294, 300, 310, 320, 330, 335, 327, 316, 304, 287, 268, 238, 228, 219, 217, 213, 210, 208, 211, 216, 221, 212, 205, 198, 185, 173, 161, 155, 140, 129, 123, 118, 115, 118, 124, 130, 138, 146, 152, 159, 161, 160, 157, 154, 153, 152, 155, 155, 152, 145, 137, 127, 115, 106, 103, 105, 109, 116, 124, 131, 138, 141, 140, 134, 129, 113, 102, 95, 95, 89, 92, 96, 102, 109, 115, 120, 125, 129, 130, 132, 137, 140, 144, 148, 151, 159, 167, 179, 193, 207, 224, 238, 246, 250, 252, 252, 251, 250, 250, 259, 270, 286, 303, 316, 323, 328, 327, 323, 316, 312, 308, 307, 309, 315, 323, 334, 344, 356, 364, 373, 378, 379, 379, 379, 376, 374, 372, 371, 370, 367, 366, 368, 372, 372, 375, 380, 382, 384, 385, 386, 385, 382, 380, 378, 373, 368, 365, 364, 364, 366, 368, 372, 375, 376, 381, 382, 380, 375, 368, 359, 349, 335, 321, 314, 303, 291, 284, 281, 281, 283, 285, 290, 293, 295, 296, 297, 297, 300, 300, 297, 299, 301, 303, 308, 310, 315, 317, 318, 323, 325, 326, 330, 333, 334, 335, 337, 337, 341, 344, 347, 349, 350, 350, 353, 355, 357, 356, 354, 349, 345, 342, 338, 333, 324, 320, 322, 321, 320, 319, 317, 311, 300, 295, 285, 269, 252, 242, 234, 223, 214, 210, 207, 206, 206, 207, 206, 209, 213, 215, 218, 219, 214, 210, 202, 195, 185, 175, 169, 163, 161, 158, 159, 159, 160, 162, 163, 162, 164, 166, 166, 167, 169, 167, 170, 167, 165, 165, 167, 172, 179, 186, 191, 199, 202, 210, 214, 217, 217, 216, 214, 213, 213, 213, 213, 215, 219, 222, 228, 236, 244, 252, 258, 262, 263, 264, 265, 268, 271, 278, 284, 293, 300, 308, 311, 313, 314, 317, 309, 308, 299, 303, 299, 304, 304, 305, 303, 303, 299, 294, 292, 289, 284, 281, 274, 274, 275, 275, 277, 279, 280, 282, 284, 281, 276, 277, 273, 269, 267, 261, 256, 256, 252, 248, 244, 247, 247, 244, 249, 256, 264, 272, 282, 290, 301, 302, 299, 294, 295, 294, 296, 303, 313, 323, 333, 343, 353, 360, 367, 371, 376, 378, 375, 375, 374, 375, 375, 374, 374, 373, 374, 375, 379, 382, 385, 388, 396, 395, 397, 396, 394, 390, 383, 374, 365, 357, 346, 339, 336, 333, 331, 333, 329, 335, 339, 345, 352, 359, 365, 370, 371, 371, 373, 368, 364, 358, 352, 346, 340, 337, 333, 333, 335, 338, 343, 353, 360, 362, 364, 363, 361, 353, 342, 332, 321, 315, 309, 311, 314, 316, 327, 329, 336, 342, 347, 343, 338, 329, 317, 307, 296, 279, 272, 263, 257, 249, 253, 256, 261, 270, 282, 296, 305, 312, 319, 319, 311, 302, 292, 278, 265, 252, 242, 236, 237, 237, 244, 254, 271, 284, 297, 308, 317, 314, 311, 303, 295, 287, 277, 268, 262, 262, 260, 267, 274, 284, 297, 308, 319, 328, 331, 333, 332, 326, 320, 312, 302, 294, 287, 289, 291, 290, 295, 302, 311, 313, 319, 324, 322, 322, 321, 319, 315, 312, 309, 307, 303, 301, 299, 297, 298, 302, 304, 306, 306, 314, 321, 327, 330, 335, 334, 335, 334, 330, 329, 327, 326, 324, 322, 320, 318, 317, 317, 321, 319, 325, 328, 330, 333, 334, 334, 334, 333, 329, 322, 318, 311, 305, 299, 297, 295, 294, 293, 290, 291, 293, 293, 292, 290, 291, 292, 293, 294, 296, 295, 291, 290, 284, 279, 273, 268, 262, 257, 253, 249, 252, 250, 254, 264, 276, 289, 298, 307, 313, 312, 314, 307, 299, 289, 280, 271, 262, 254, 251, 246, 243, 236, 237, 232, 227, 224, 221, 218, 215, 208, 208, 206, 206, 204, 209, 215, 221, 231, 236, 241, 245, 251, 258, 265, 273, 277, 281, 287, 293, 298, 302, 307, 313, 317, 323, 322, 323, 328, 335, 340, 349, 348, 349, 349, 346, 342, 338, 332, 325, 322, 317, 324, 330, 340, 348, 359, 370, 379, 382, 381, 384, 383, 381, 378, 374, 372, 367, 362, 360, 361, 363, 364, 366, 368, 370, 366, 359, 353, 346, 333, 329, 320, 314, 308, 301, 295, 291, 284, 278, 275, 271, 270, 269, 272, 274, 276, 277, 277, 274, 273, 271, 268, 268, 262, 261, 261, 260, 262, 264, 264, 264, 262, 258, 252, 246, 238, 231, 222, 215, 211, 206, 203, 204, 203, 201, 196, 194, 190, 189, 181, 182, 182, 181, 184, 191, 200, 211, 223, 236, 248, 257, 261, 264, 263, 261, 259, 254, 253, 254, 260, 269, 279, 290, 300, 310, 320, 325, 328, 329, 328, 327, 325, 324, 324, 327, 331, 337, 343, 350, 355, 360, 362, 361, 360, 353, 346, 339, 331, 322, 317, 315, 317, 318, 319, 321, 324, 329, 328, 329, 332, 327, 323, 318, 309, 303, 295, 285, 277, 272, 269, 268, 272, 279, 293, 303, 314, 325, 335, 345, 346, 338, 326, 316, 305, 295, 286, 280, 279, 285, 291, 296, 302, 307, 308, 308, 307, 302, 304, 298, 292, 290, 290, 296, 301, 308, 313, 315, 316, 311, 305, 298, 290, 284, 278, 272, 269, 269, 267, 266, 265, 270, 277, 285, 294, 305, 316, 325, 330, 331, 328, 327, 318, 302, 296, 286, 287, 285, 293, 302, 311, 321, 332, 339, 345, 347, 344, 343, 337, 334, 332, 329, 331, 332, 334, 341, 350, 359, 365, 368, 372, 371, 368, 365, 360, 357, 357, 356, 357, 360, 361, 365, 361, 362, 355, 345, 333, 323, 311, 304, 296, 291, 285, 283, 284, 291, 292, 297, 302, 307, 312, 315, 317, 318, 316, 315, 308, 301, 296, 291, 291, 289, 287, 293, 299, 311, 322, 334, 345, 354, 355, 353, 349, 344, 336, 326, 318, 312, 311, 317, 323, 331, 338, 346, 351, 356, 352, 350, 344, 334, 324, 315, 307, 304, 301, 301, 306, 312, 315, 320, 323, 326, 329, 327, 326, 324, 317, 308, 302, 296, 296, 291, 292, 296, 303, 310, 317, 319, 324, 321, 320, 318, 316, 311, 307, 301, 297, 296, 297, 305, 310, 315, 321, 332, 335, 333, 332, 328, 321, 314, 308, 299, 293, 289, 289, 290, 293, 296, 297, 297, 295, 287, 280, 273, 267, 261, 254, 250, 246, 245, 244, 247, 256, 259, 269, 277, 284, 286, 283, 280, 277, 269, 266, 266, 265, 272, 280, 293, 304, 320, 331, 338, 344, 342, 336, 329, 323, 323, 326, 335, 344, 353, 360, 368, 374, 374, 373, 368, 362, 358, 358, 359, 362, 365, 367, 369, 369, 373, 375, 378, 382, 385, 388, 395, 395, 400, 403, 401, 399, 393, 388, 383, 379, 378, 379, 379, 378, 375, 367, 364, 359, 353, 348, 348, 347, 348, 349, 349, 349, 346, 341, 338, 328, 319, 310, 304, 299, 297, 294, 295, 298, 301, 306, 311, 317, 323, 329, 332, 330, 323, 319, 314, 312, 309, 315, 322, 332, 342, 352, 363, 372, 379, 382, 383, 384, 384, 381, 380, 378, 377, 376, 377, 376, 376, 378, 380, 384, 387, 389, 391, 393, 394, 394, 392, 391, 390, 390, 390, 389, 390, 392, 395, 398, 401, 403, 403, 400, 398, 395, 391, 392, 382, 378, 376, 374, 373, 372, 372, 373, 375, 378, 380, 382, 383, 380, 375, 368, 363, 358, 354, 348, 343, 343, 344, 344, 347, 355, 355, 360, 366, 370, 376, 380, 381, 378, 376, 371, 366, 360, 355, 353, 352, 350, 348, 345, 342, 340, 343, 343, 342, 346, 343, 345, 346, 344, 340, 335, 328, 322, 315, 309, 303, 298, 293, 287, 286, 290, 292, 297, 305, 311, 321, 328, 333, 337, 342, 337, 333, 328, 321, 314, 306, 302, 304, 311, 321, 328, 341, 349, 361, 373, 374, 375, 375, 373, 369, 363, 359, 353, 348, 343, 337, 336, 337, 337, 334, 331, 330, 327, 326, 320, 319, 321, 313, 310, 302, 293, 282, 275, 267, 258, 251, 246, 245, 248, 252, 262, 275, 285, 297, 306, 312, 319, 321, 323, 318, 315, 308, 305, 311, 312, 323, 334, 347, 359, 371, 379, 384, 385, 378, 369, 359, 350, 342, 337, 335, 335, 341, 346, 352, 360, 364, 368, 368, 365, 359, 351, 339, 330, 320, 309, 301, 297, 291, 291, 292, 299, 299, 304, 310, 314, 320, 325, 330, 332, 331, 331, 323, 319, 313, 313, 319, 324, 331, 338, 344, 350, 354, 354, 352, 349, 345, 342, 337, 332, 329, 328, 326, 325, 326, 328, 332, 333, 339, 336, 334, 331, 325, 316, 309, 298, 289, 282, 276, 275, 275, 277, 282, 286, 292, 295, 296, 293, 288, 282, 271, 265, 256, 247, 242, 239, 238, 240, 243, 247, 252, 258, 265, 271, 279, 285, 293, 298, 305, 309, 311, 310, 311, 309, 305, 301, 302, 312, 322, 335, 349, 363, 371, 372, 371, 368, 365, 361, 358, 360, 364, 374, 382, 389, 398, 402, 401, 396, 387, 383, 371, 362, 356, 353, 354, 352, 355, 354, 353, 349, 341, 332, 323, 316, 313, 309, 307, 306, 310, 310, 307, 302, 296, 288, 282, 276, 271, 268, 265, 262, 263, 265, 269, 274, 281, 277, 276, 273, 263, 255, 249]
  out "LIVE":bool
  in  "stop":bool
  out "Camera backlog":i32(slide)=-1 scale=0.0..50.0
  in  "IMAQdx Device Camera":T3="cam2"
  in  "Buffers Camera 1":u32=50
  out "Image":T4(plugin-control)
  # "PROGRAM INFO\n\nThis program finds the\nfirst pixel below the \nuser threshold in\nthe user specified\nROI below"
  # "Camera search ROI"
  # "Data acquisition \nsettings"
  # "issues\n\nHow do we know if frames \nare dropped?\n\nProbably will need to save data\nin sections to an open file\n\nCould have a sliding ROI based\non previous trailing edge position\n\nCould process each data chunk\nseparately to avoid frame dropping\nissues.  I.e. if you write every 1000\npoints, then in post processing only\nprocess 1000 at a time."
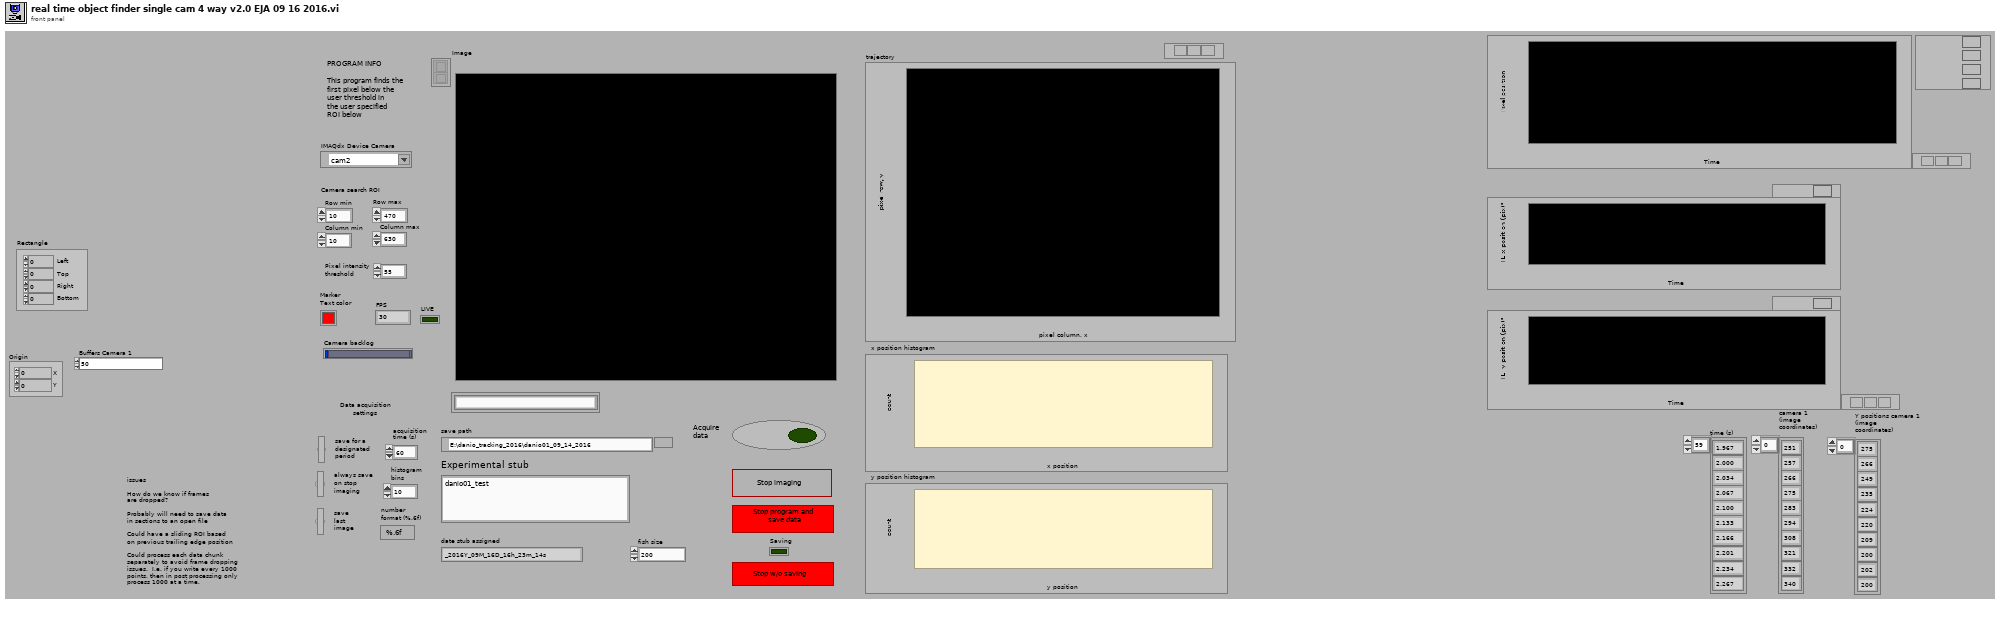
[diagram p1: front panel]
types:
  T1 = cluster{"Left":i32, "Top":i32, "Right":i32, "Bottom":i32}
  T2 = cluster{"X Values":dbl[], "Histogram: h(x)":i32[]}
  T3 = typedef "IMAQdx.ctl" = refnum<k21>
  T4 = typedef "IMAQ Image.ctl" = refnum<image>
  T5 = typedef "NI_Vision_Acquisition_Software.lvlib/IMAQdx Buffer Number Mode.ctl" = enum32{"Next", "Last", "Buffer Number"}
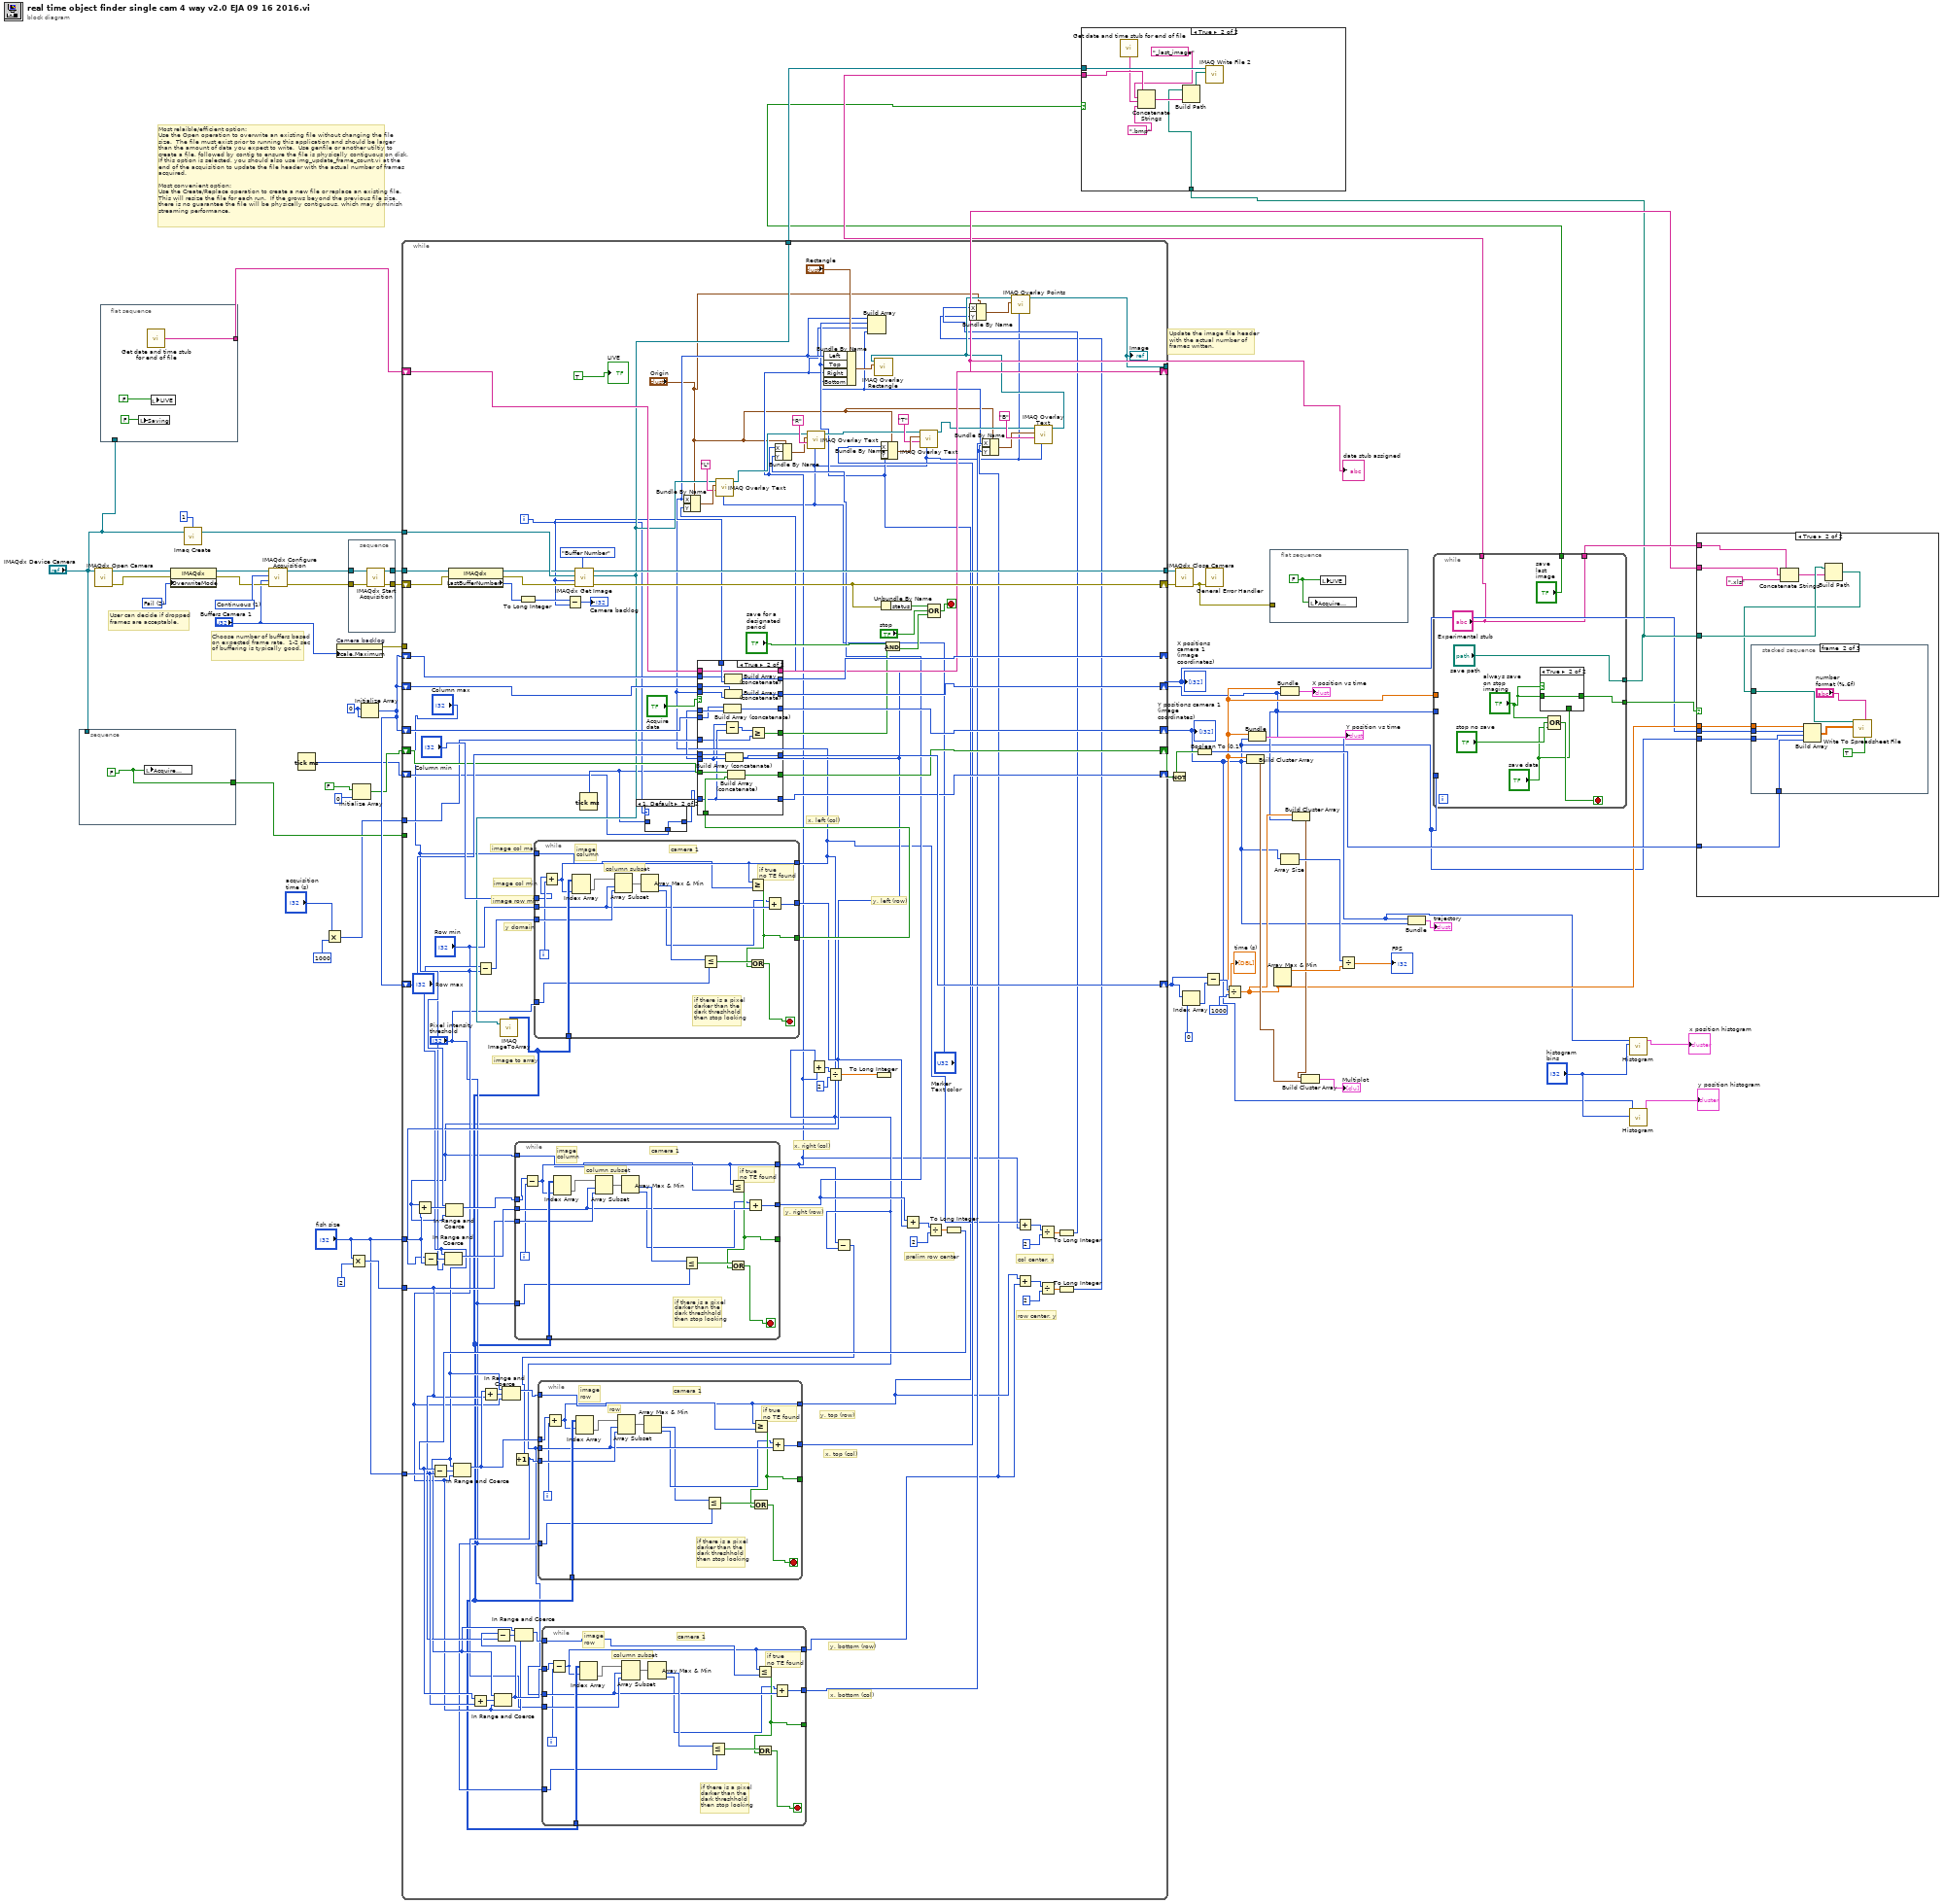
[diagram p0: block diagram]
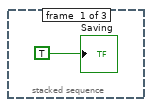
[diagram p4: hidden frame]
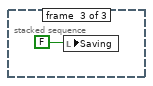
[diagram p5: hidden frame]
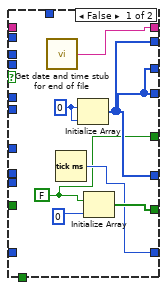
[diagram p8: hidden frame]
diagram:
  w31 = 0
  w55 = u32 2 items=["Get Oldest"=0, "Fail"=2, "Get Newest"=3] ("OverwriteMode")
  w61 = u32 1 items=["One Shot", "Continuous"] ("Continuous ?")
  # "Update the image file header with the actual number of frames written."
  # "Choose number of buffers based on expected frame rate.  1-2 sec of buffering is typically good."
  # "User can decide if dropped frames are acceptable."
  # "Most relaible/efficient option:\nUse the Open operation to overwrite an existing file without changing the file size.  The file must exist prior to running this application and should be larger than the amount of data you expect to write.  Use genfile or another utiltiy to create a file, followed by contig to ensure the file is physically contiguous on disk.  If this option is selected, you should also use img_update_frame_count.vi at the end of the acquisition to update the file header with the actual number of frames acquired. \n\nMost convenient option:\nUse the Create/Replace operation to create a new file or replace an existing file. This will resize the file for each run.  If the grows beyond the previous file size, there is no guarantee the file will be physically contiguous, which may diminish streaming performance."
  n1 = stacked-sequence {
    tunnel: "IMAQdx Device Camera" -> [_]
    tunnel: [w63] -> w15
    frame #0 {
      w63 = FALSE
      n2 = local write "Acquire\ndata"(w63) -> ()
    }
  }
  n3 = call <vilib>:"IMAQdx Open Camera.vi"("Session In"="IMAQdx Device Camera") -> ("error out"=w51:errorcluster, "Session Out"=w50:T3)  [unwired: 2 in, 7 out]
  n4 = flat-sequence {
    tunnel: "IMAQdx Device Camera" -> [_]
    tunnel: [w64] -> w30
    frame #0 {
      n5 = local write "Saving"(FALSE) -> ()
      n6 = call <userlib>:"Get date and time stub for end of file.vi"() -> ("date and time stub"=w64:string)
      n7 = local write "LIVE"(FALSE) -> ()
    }
  }
  n8 = property class="IMAQdx"(reference=w50, error in=w51, "OverwriteMode"=w55) -> (reference out=w53:T3, error out=w52:errorcluster)
  n9 = call "Imaq Create"("Border Size"=1, "Image Name"="IMAQdx Device Camera") -> ("New Image"=w62:T4)  [unwired: 2 in, 2 out]
  n10 = call <vilib>:"IMAQdx Configure Acquisition.vi"("error in"=w52, "Number of Buffers"="Buffers Camera 1", "Continuous?"=w61, "Session In"=w53) -> ("error out"=w47:errorcluster, "Session Out"=w54:T3)  [unwired: 6 out]
  n11 = Tick Count (ms)() -> (millisecond timer value=w9:u32)
  n12 = Multiply(x="acquisition \ntime (s)", y=1000) -> (x*y=w10:i32)
  n13 = property on="Camera backlog" class="Slide (strict)"("Scale.Maximum"="Buffers Camera 1") -> (error out=w49:errorcluster)  [unwired: 2 in, 1 out]
  n14 = stacked-sequence {
    tunnel: [w70] -> w60
    tunnel: [w69] -> w59
    tunnel: w54 -> [w68]
    tunnel: w47 -> [w67]
    frame #0 {
      n15 = call <vilib>:"IMAQdx Start Acquisition.vi"("error in"=w67, "Session In"=w68) -> ("error out"=w70:errorcluster, "Session Out"=w69:T3)  [unwired: 8 out]
    }
  }
  n16 = Multiply(x="fish size", y=2) -> (x*y=w2:i32)
  n17 = Initialize Array(FALSE, 0) -> (w22:bool[])
  n18 = Initialize Array(w31, w31) -> (w28:i32[])
  n19 = while {
    tunnel: [w169] -> w57
    tunnel: w59 -> [w172]
    tunnel: w62 -> [w170]
    tunnel: [w71] -> _
    shift-right: [w168] -> w56
    shift-left: w60 -> [w171]
    tunnel: w49 -> [_]
    shift-right: [w153] -> _
    shift-left: w28 -> [w154]
    shift-right: [w152] -> w8
    shift-left: w28 -> [w151]
    shift-right: [w150] -> w4
    shift-left: w28 -> [w149]
    shift-right: [w148] -> w41
    shift-left: w28 -> [w147]
    shift-right: [w145] -> w29
    shift-left: w30 -> [w146]
    shift-right: [w143] -> w27
    shift-left: w22 -> [w144]
    tunnel: [w141] -> w20
    tunnel: w15 -> [_]
    shift-right: [w140] -> _
    shift-left: w9 -> [w132]
    tunnel: w10 -> [w139]
    tunnel: "fish size" -> [w128]
    tunnel: w2 -> [w102]
    tunnel: "fish size" -> [w105]
    i -> [w135]
    stop <- w174 stop-if-true
    # "x, top (col)"
    # "y, top (row)"
    # "row center, y"
    # "col center, x"
    # "y, bottom (row)"
    # "x, bottom (col)"
    # "prelim row center"
    # "x, right (col)"
    # "y, right (row)"
    # "image col min"
    # "image col max"
    # "image row min"
    # "y, left (row)"
    # "x, left (col)"
    # "y domain"
    # "image to array"
    n20 = property class="IMAQdx"(reference=w172, error in=w171) -> (reference out=w165:T3, error out=w166:errorcluster, "LastBufferNumber"=w162:u32)
    n21 = Subtract(x="Row max", y="Row min") -> (x-y=w156:i32)
    n22 = To Long Integer(number=w162) -> (32bit integer=w161:i32)
    n23 = Subtract(x=w161, y=w135) -> (x-y=→"Camera backlog":i32)
    n24 = call <vilib>:"IMAQdx Get Image.vi"("Buffer Number Mode (Next)"=IMAQdx_Buffer_Number_Mode."Buffer Number", "error in"=w166, "Buffer Number In"=w135, "Image In"=w170, "Session In"=w165) -> ("error out"=w168:errorcluster, "Image Out"=w141:T4, "Session Out"=w169:T3)  [unwired: 1 in, 3 out]
    n25 = call "IMAQ ImageToArray"("Image"=w141) -> ("Image Pixels (U8)"=w95:u8[][])  [unwired: 2 in, 5 out]
    n26 = while {
      tunnel: "Row min" -> [w261]
      tunnel: [w260] -> w81
      tunnel: [w262] -> w115
      tunnel: w156 -> [w264]
      tunnel: w95 -> [w266]
      tunnel: "Column max" -> [w252]
      tunnel: "Column min" -> [w253]
      tunnel: [w257] -> w142
      tunnel: "Pixel intensity\nthreshold" -> [w255]
      i -> [w254]
      stop <- w258 stop-if-true
      # "if true\nno TE found"
      # "camera 1"
      # "if there is a pixel\ndarker than the\ndark threshhold\nthen stop looking"
      # "column subset"
      # "image\ncolumn"
      n27 = Add(x=w253, y=w254) -> (x+y=w260:i32)
      n28 = Index Array(array=w266, index (col)=w260) -> (element=w265:u8[])  [unwired: 1 in]
      n29 = Array Subset(array=w265, index=w261, length=w264) -> (w263:u8[])
      n30 = Array Max & Min(array=w263) -> (min value=w267:u8, min index (indices)=w256:i32)  [unwired: 2 out]
      n31 = Less Or Equal?(x=w267, y=w255) -> (x <= y?=w259:bool)
      n32 = Greater Or Equal?(x=w260, y=w252) -> (x >= y?=w257:bool)
      n33 = Or(x=w259, y=w257) -> (x .or. y?=w258:bool)
      n34 = Add(x=w256, y=w261) -> (x+y=w262:i32)
    }
    n35 = Add(x=w81, y=w128) -> (x+y=w131:i32)
    n36 = Subtract(x=w115, y=w128) -> (x-y=w127:i32)
    n37 = In Range and Coerce(upper limit="Row max", x=w127, lower limit="Row min") -> (coerced(x)=w126:i32)  [unwired: 1 out]
    n38 = In Range and Coerce(upper limit="Column max", x=w131, lower limit=w81) -> (coerced(x)=w129:i32)  [unwired: 1 out]
    n39 = while {
      tunnel: w126 -> [w216]
      tunnel: [w215] -> w79
      tunnel: [w217] -> w116
      tunnel: w102 -> [w219]
      tunnel: w95 -> [w221]
      tunnel: w81 -> [w207]
      tunnel: w129 -> [w208]
      tunnel: [w212] -> _
      tunnel: "Pixel intensity\nthreshold" -> [w210]
      i -> [w209]
      stop <- w213 stop-if-true
      # "if true\nno TE found"
      # "camera 1"
      # "if there is a pixel\ndarker than the\ndark threshhold\nthen stop looking"
      # "column subset"
      # "image\ncolumn"
      n40 = Subtract(x=w208, y=w209) -> (x-y=w215:i32)
      n41 = Index Array(array=w221, index (col)=w215) -> (element=w220:u8[])  [unwired: 1 in]
      n42 = Array Subset(array=w220, index=w216, length=w219) -> (w218:u8[])
      n43 = Array Max & Min(array=w218) -> (min value=w222:u8, min index (indices)=w211:i32)  [unwired: 2 out]
      n44 = Less Or Equal?(x=w222, y=w210) -> (x <= y?=w214:bool)
      n45 = Less Or Equal?(x=w215, y=w207) -> (x <= y?=w212:bool)
      n46 = Or(x=w214, y=w212) -> (x .or. y?=w213:bool)
      n47 = Add(x=w211, y=w216) -> (x+y=w217:i32)
    }
    n48 = Tick Count (ms)() -> (millisecond timer value=w134:u32)
    n49 = case shown="1, Default" w135 {
      tunnel: w134 -> [w223 _]
      tunnel: [w223 w224] -> w133
      tunnel: w132 -> [_ w224]
      frame 0 {
      }
      frame 1, Default {
      }
    }
    n50 = Bundle By Name(cluster="Origin", "X"=w81, "Y"=w115) -> (w159:cluster{"X":i32, "Y":i32})
    n51 = case shown="True" "Acquire\ndata" {
      tunnel: w135 -> [_ w251]
      tunnel: w154 -> [_ w250]
      tunnel: [w229 w249] -> w153
      tunnel: w81 -> [_ w247]
      tunnel: [w229 w248] -> w152
      tunnel: w151 -> [_ w246]
      tunnel: w115 -> [_ w245]
      tunnel: [w229 w244] -> w150
      tunnel: w149 -> [_ w243]
      tunnel: w134 -> [_ w235]
      tunnel: [w229 w242] -> w148
      tunnel: w147 -> [_ w241]
      tunnel: [w230 w240] -> w145
      tunnel: w146 -> [_ w240]
      tunnel: w144 -> [_ w239]
      tunnel: w142 -> [_ w238]
      tunnel: [w227 w237] -> w143
      tunnel: w133 -> [_ w234]
      tunnel: [w226 w234] -> w140
      tunnel: w139 -> [_ w233]
      tunnel: [w225 w232] -> w138
      frame False {
        w225 = FALSE
        w231 = 0
        n52 = call <userlib>:"Get date and time stub for end of file.vi"() -> ("date and time stub"=w230:string)
        n53 = Tick Count (ms)() -> (millisecond timer value=w226:u32)
        n54 = Initialize Array(w231, w231) -> (w229:i32[])
        n55 = Initialize Array(w225, 0) -> (w227:bool[])
      }
      frame True {
        n56 = Subtract(x=w235, y=w234) -> (x-y=w236:u32)
        n57 = Build Array (concatenate)(w243, w245) -> (w244:i32[])
        n58 = Build Array (concatenate)(w250, w251) -> (w249:i32[])
        n59 = Build Array (concatenate)(w246, w247) -> (w248:i32[])
        n60 = Build Array (concatenate)(w241, w235) -> (w242:u32[])
        n61 = Build Array (concatenate)(w239, w238) -> (w237:bool[])
        n62 = Greater Or Equal?(x=w236, y=w233) -> (x >= y?=w232:bool)
      }
    }
    n63 = call "IMAQ Overlay Text"("Text Color (black)"="Marker\nText color", "String"="L", "Origin"=w159, "Image"=w141) -> ("Image Out"=w123:T4)  [unwired: 4 in, 3 out]
    n64 = Bundle By Name(cluster="Origin", "X"=w79, "Y"=w116) -> (w124:cluster{"X":i32, "Y":i32})
    n65 = call "IMAQ Overlay Text"("Text Color (black)"="Marker\nText color", "String"="R", "Origin"=w124, "Image"=w123) -> ("Image Out"=w108:T4)  [unwired: 4 in, 3 out]
    n66 = Add(x=w81, y=w79) -> (x+y=w122:i32)
    n67 = Divide(x=w122, y=2) -> (x/y=w120:dbl)
    n68 = Subtract(x=w79, y=w81) -> (x-y=w98:i32)
    n69 = Increment(x=w98) -> (x+1=w97:i32)
    n70 = To Long Integer(number=w120) -> ()  [unwired: 1 out]
    n71 = Unbundle By Name(w168) -> ("status"=w173:bool)
    n72 = And(x="save for a \ndesignated \nperiod", y=w138) -> (x .and. y?=w137:bool)
    n73 = Add(x=w116, y=w115) -> (x+y=w117:i32)
    n74 = Divide(x=w117, y=2) -> (x/y=w119:dbl)
    n75 = Compound Arithmetic op=OR(w173, "stop", w137) -> (w174:bool)
    n76 = To Long Integer(number=w119) -> (32bit integer=w106:i32)
    n77 = Subtract(x=w106, y=w105) -> (x-y=w114:i32)
    n78 = In Range and Coerce(upper limit="Row max", x=w114, lower limit="Row min") -> (coerced(x)=w113:i32)  [unwired: 1 out]
    n79 = Add(x=w106, y=w105) -> (x+y=w107:i32)
    n80 = Add(x=w113, y=w102) -> (x+y=w112:i32)
    n81 = In Range and Coerce(upper limit="Row max", x=w107, lower limit="Row min") -> (coerced(x)=w103:i32)  [unwired: 1 out]
    n82 = Subtract(x=w103, y=w102) -> (x-y=w104:i32)
    n83 = In Range and Coerce(upper limit="Row max", x=w112, lower limit="Row min") -> (coerced(x)=w111:i32)  [unwired: 1 out]
    n84 = In Range and Coerce(upper limit="Row max", x=w104, lower limit="Row min") -> (coerced(x)=w99:i32)  [unwired: 1 out]
    n85 = while {
      tunnel: w81 -> [w201]
      tunnel: [w192] -> w80
      tunnel: [w202] -> w94
      tunnel: w97 -> [w204]
      tunnel: w95 -> [w206]
      tunnel: w111 -> [w193]
      tunnel: w113 -> [w194]
      tunnel: [w198] -> _
      tunnel: "Pixel intensity\nthreshold" -> [w196]
      i -> [w195]
      stop <- w199 stop-if-true
      # "if true\nno TE found"
      # "camera 1"
      # "if there is a pixel\ndarker than the\ndark threshhold\nthen stop looking"
      # "row"
      # "image row"
      n86 = Add(x=w194, y=w195) -> (x+y=w192:i32)
      n87 = Index Array(array=w206, index (row)=w192) -> (element=w205:u8[])  [unwired: 1 in]
      n88 = Array Subset(array=w205, index=w201, length=w204) -> (w203:u8[])
      n89 = Array Max & Min(array=w203) -> (min value=w191:u8, min index (indices)=w197:i32)  [unwired: 2 out]
      n90 = Less Or Equal?(x=w191, y=w196) -> (x <= y?=w200:bool)
      n91 = Greater Or Equal?(x=w192, y=w193) -> (x >= y?=w198:bool)
      n92 = Or(x=w200, y=w198) -> (x .or. y?=w199:bool)
      n93 = Add(x=w197, y=w201) -> (x+y=w202:i32)
    }
    n94 = while {
      tunnel: w81 -> [w184]
      tunnel: [w175] -> w78
      tunnel: [w185] -> w90
      tunnel: w97 -> [w187]
      tunnel: w95 -> [w189]
      tunnel: w99 -> [w176]
      tunnel: w103 -> [w177]
      tunnel: [w181] -> _
      tunnel: "Pixel intensity\nthreshold" -> [w179]
      i -> [w178]
      stop <- w182 stop-if-true
      # "if true\nno TE found"
      # "camera 1"
      # "if there is a pixel\ndarker than the\ndark threshhold\nthen stop looking"
      # "column subset"
      # "image row"
      n95 = Subtract(x=w177, y=w178) -> (x-y=w175:i32)
      n96 = Index Array(array=w189, index (row)=w175) -> (element=w188:u8[])  [unwired: 1 in]
      n97 = Array Subset(array=w188, index=w184, length=w187) -> (w186:u8[])
      n98 = Array Max & Min(array=w186) -> (min value=w190:u8, min index (indices)=w180:i32)  [unwired: 2 out]
      n99 = Less Or Equal?(x=w190, y=w179) -> (x <= y?=w183:bool)
      n100 = Less Or Equal?(x=w175, y=w176) -> (x <= y?=w181:bool)
      n101 = Or(x=w183, y=w181) -> (x .or. y?=w182:bool)
      n102 = Add(x=w180, y=w184) -> (x+y=w185:i32)
    }
    n103 = Bundle By Name(cluster="Rectangle", "Left"=w81, "Top"=w80, "Right"=w79, "Bottom"=w78) -> (w88:T1)
    n104 = Build Array(w81, w80, w79, w78) -> ()  [unwired: 1 out]
    n105 = Bundle By Name(cluster="Origin", "X"=w94, "Y"=w80) -> (w110:cluster{"X":i32, "Y":i32})
    n106 = call "IMAQ Overlay Text"("Text Color (black)"="Marker\nText color", "String"="T", "Origin"=w110, "Image"=w108) -> ("Image Out"=w91:T4)  [unwired: 4 in, 3 out]
    n107 = Bundle By Name(cluster="Origin", "X"=w90, "Y"=w78) -> (w92:cluster{"X":i32, "Y":i32})
    n108 = Add(x=w81, y=w79) -> (x+y=w87:i32)
    n109 = Add(x=w80, y=w78) -> (x+y=w82:i32)
    n110 = call "IMAQ Overlay Text"("Text Color (black)"="Marker\nText color", "String"="B", "Origin"=w92, "Image"=w91) -> ("Image Out"=w77:T4)  [unwired: 4 in, 3 out]
    n111 = call "IMAQ Overlay Rectangle"("Rectangle"=w88, "Image"=w77) -> ()  [unwired: 8 in, 2 out]
    n112 = Divide(x=w87, y=2) -> (x/y=w85:dbl)
    n113 = Divide(x=w82, y=2) -> (x/y=w84:dbl)
    n114 = To Long Integer(number=w85) -> (32bit integer=w74:i32)
    n115 = To Long Integer(number=w84) -> (32bit integer=w73:i32)
    n116 = Bundle By Name(cluster="Origin", "X"=w74, "Y"=w73) -> (w76:cluster{"X":i32, "Y":i32})
    n117 = call "IMAQ Overlay Points"("Color"="Marker\nText color", "Point"=w76, "Image"=w77) -> ("Image Out"=w71:T4)  [unwired: 7 in, 1 out]
    "Image" <- w71
    "LIVE" <- TRUE
  }
  "X positions\ncamera 1\n(image \ncoordinates)" <- w8
  "Y positions camera 1 \n(image \ncoordinates)" <- w4
  "date stub assigned" <- w29
  n118 = Not(x=w27) -> (.not. x?=w24:bool[])
  n119 = call <vilib>:"IMAQdx Close Camera.vi"("error in"=w56, "Session In"=w57) -> ("error out"=w46:errorcluster)  [unwired: 9 out]
  n120 = Index Array(array=w41, index=0) -> (element=w42:u32)
  n121 = Boolean To (0,1)(Boolean=w24) -> (0, 1=w23:i16[])
  n122 = Subtract(x=w41, y=w42) -> (x-y=w36:u32[])
  n123 = call <vilib>:"General Error Handler.vi"("error in (no error)"=w46) -> ()  [unwired: 1 in, 14 out]
  n124 = Divide(x=w36, y=1000) -> (x/y=w14:dbl[])
  "time (s)" <- w14
  n125 = Build Cluster Array(w14, w4) -> (w33:cluster{dbl, i32}[])
  n126 = Bundle(w14, w4) -> (→"Y position vs time":cluster{dbl[], i32[]})  [unwired: 1 out]
  n127 = flat-sequence {
    tunnel: w46 -> [_]
    frame #0 {
      w268 = FALSE
      n128 = local write "Acquire\ndata"(w268) -> ()
      n129 = local write "LIVE"(w268) -> ()
    }
  }
  n130 = Array Max & Min(array=w14) -> (max value=w40:dbl)  [unwired: 3 out]
  n131 = Bundle(w14, w8) -> (→"X position vs time":cluster{dbl[], i32[]})  [unwired: 1 out]
  n132 = Array Size(array=w4) -> (size(s)=w39:i32)
  n133 = Build Cluster Array(w14, w8) -> (w34:cluster{dbl, i32}[])
  n134 = Build Cluster Array(w34, w33) -> (→"Multiplot":cluster{cluster{dbl, i32}[]}[])
  n135 = Divide(x=w39, y=w40) -> (x/y=→"FPS":dbl)
  n136 = Bundle(w8, w4) -> (→"trajectory":cluster{i32[], i32[]})  [unwired: 1 out]
  n137 = while {
    tunnel: w14 -> [_]
    tunnel: w8 -> [_]
    tunnel: w4 -> [_]
    tunnel: ["save path"] -> w18
    tunnel: ["Experimental stub"] -> w32
    tunnel: [w270] -> w21
    tunnel: ["Experimental stub"] -> w19
    tunnel: ["save\nlast\nimage"] -> w17
    stop <- w272 stop-if-true
    n138 = case shown="True" "always save\non stop\nimaging" {
      tunnel: [w277 w278] -> w270
      tunnel: "always save\non stop\nimaging" -> [_ w278]
      tunnel: "save data" -> [w277 _]
      frame False {
      }
      frame True {
      }
    }
    n139 = Compound Arithmetic op=OR("always save\non stop\nimaging", "stop no save", "save data") -> (w272:bool)
  }
  n140 = case shown="True" w17 {
    tunnel: w20 -> [_ w286]
    tunnel: w19 -> [_ w284]
    tunnel: w18 -> [_ w279]
    frame False {
    }
    frame True {
      n141 = call <userlib>:"Get date and time stub for end of file.vi"() -> ("date and time stub"=w282:string)
      n142 = Concatenate Strings(w284, "_last_image", w282, ".bmp") -> (w285:string)
      n143 = Build Path(base path=w279, name or relative path=w285) -> (appended path=w280:path)
      n144 = call-poly "IMAQ Write File 2"("File Path"=w280, "Image"=w286) -> ()  [unwired: 8 in, 2 out]
    }
  }
  n145 = call <vilib>:"Histogram.vi"("intervals"="histogram \nbins", "X"=w8) -> ("Histogram Graph"=→"x position histogram":T2)  [unwired: 6 in, 3 out]
  n146 = call <vilib>:"Histogram.vi"("intervals"="histogram \nbins", "X"=w4) -> ("Histogram Graph"=→"y position histogram":T2)  [unwired: 6 in, 3 out]
  n147 = case shown="True" w21 {
    tunnel: w14 -> [_ w296]
    tunnel: w8 -> [_ w295]
    tunnel: w4 -> [_ w294]
    tunnel: w32 -> [_ w292]
    tunnel: w18 -> [_ w291]
    tunnel: w29 -> [_ w288]
    tunnel: w23 -> [_ w287]
    frame False {
    }
    frame True {
      n148 = Concatenate Strings(w292, w288, ".xls") -> (w290:string)
      n149 = Build Path(base path=w291, name or relative path=w290) -> (appended path=w289:path)
      n150 = stacked-sequence {
        tunnel: w289 -> [_ w303 _]
        tunnel: w296 -> [_ w302 _]
        tunnel: w295 -> [_ w301 _]
        tunnel: w294 -> [_ w300 _]
        tunnel: w287 -> [_ w299 _]
        frame #0 {
          "Saving" <- TRUE
        }
        frame #1 {
          n151 = Build Array(w302, w301, w300, w299) -> (w298:dbl[][])
          n152 = call-poly <vilib>:"Write To Spreadsheet File.vi"("transpose? (no:F)"=TRUE, "format (%.3f)"="number\nformat (%.6f)", "2D data"=w298, "file path (dialog if empty)"=w303) -> ()  [unwired: 4 in, 1 out]
        }
        frame #2 {
          n153 = local write "Saving"(FALSE) -> ()
        }
      }
    }
  }
